vi "InVivoComputationalCannulaMicroscopeVi_v3.vi"() -> ()   [LabVIEW 2016]
doc: "The Grab and Attributes Setup example VI allows the user to view the current attributes and settings, update attribute settings, acquire images continuously, and display the images in an image control."
uses:
  <vilib>/Utility/error.llb/DialogType.ctl
  IVCCM Software V2/LabView Library/APT/callback_Done.vi
  IVCCM Software V2/LabView Library/GlobalVariables.vi
  D:/amcamsdk.20210816/extras/labview/toupcam.dll
  <vilib>/vision/NI_Vision_Development_Module.lvlib
panel:
  out "imgPro":u8[][](graph)
  in  "Imaging status":u16
  out "Error Out Surf Prep 2":errorcluster
  out "Error Surf 2":errorcluster
  in  "Full Toup Resolution":bool
  out "Image 2":u8[][](graph) caption="Image"
  out "Image":u16[][](graph)
  in  "Camera Idx":i32
  in  "Color Plane":i32(ring)=1 items=["Red", "Green", "Blue", "Hue", "Saturation", "Luminance", "Value", "Intensity"]
  out "objRef":u8[][](graph)
  in  "HW Tab":T1(tab)
  in  "LightVoltage":dbl
  in  "LightValue (v)":bool
  in  "MG17MotorZ":refnum<k7>(container)
  in  "MG17MotorY":refnum<k7>(container)
  in  "MG17MotorX":refnum<k7>(container)
  in  "Light Off (0v)":bool
  in  "Light On (5v)":bool
  in  "Grab":bool
  in  "ExpoGain":u16(slide) scale=100.0..5000.0
  in  "Expotime (ms)":dbl(slide)=300.0 scale=0.1..3600000.0
  in  "Saturation":i32(slide) scale=0.0..255.0
  in  "Hue":i32(slide) scale=-180.0..180.0
  in  "Gamma":i32(slide) scale=20.0..180.0
  in  "Contrast":i32(slide) scale=-100.0..100.0
  in  "Brightness":i32(slide) scale=-64.0..64.0
  in  "Error":errorcluster
  in  "Expotime_Min":u32
  in  "Expotime_Max":u32
  in  "ExpoGain_Min":u16
  in  "ExpoGain_Max":u16
  in  "ExpoGain_def":u16
  in  "Expotime_def":u32
  in  "LED Power":dbl=0.5
  in  "Orca Crop 2048x2048":T2={"Horizontal Offset"=1100, "Vertical Offset"=900, "Horizontal Width"=700, "Vertical Width"=700}
  in  "Toup Crop 5440x3648":T2={"Horizontal Offset"=3300, "Vertical Offset"=1200, "Horizontal Width"=1200, "Vertical Width"=1200}
  out "Timestamp":dbl
  out "Frames Per Second":dbl
  out "Library Version":string
  out "DCAM Version":string
  out "Error Cal":errorcluster
  in  "Z Index":i32=1
  out "Error Out Wait":errorcluster
  out "Error Surf":errorcluster
  out "Error Out Surf Prep":errorcluster
  out "Moving...":bool
  out "Saving...":bool
  in  "Pause":bool
  in  "Play":bool
  in  "Single":bool caption="Blank Button"
  in  "Load Cal":bool
  in  "Save Data":bool
  in  "Tab Control":T3(tab)
  in  "Stop Realtime\npix2pix":bool
  in  "Start Realtime\npix2pix":bool
  in  "Orca Exposure":dbl=3.0
  in  "Masking":bool
  in  "Threshold":dbl(slide) min=0.0 max=1.0 step=0.05 scale=0.0..1.0
  in  "Brigtness":dbl(slide) min=0.0 max=1.0 step=0.05 scale=0.0..1.0
  in  "Ctrl Factor":dbl(slide)=0.1 caption="Vertical Pointer Slide" min=0.0 max=100.0 step=0.01 scale=0.01..100.0
  in  "Shift input X":dbl step=1.0 format="%#.6g"
  in  "Shift Y":dbl step=1.0
  in  "Gain":dbl(slide)=1.0 min=1.0 step=0.05 scale=1.0..5.0
  in  "Convolution":bool
  in  "Frame Ave Count":dbl=1.0 min=0.0 max=1.0
  in  "Method":enum16{"Tikhonov", "DBS", "TSVD"}(ring)
  in  "Workspace":path=path "C:/Hun/Data/Calibration"
  in  "Kinetic Series":bool
  in  "Mask size (%)":i32=100 min=10 max=100 step=1
  in  "Mask Shift X":i32
  in  "Mask Shift Y":i32
  in  "Save image for pix2pix":bool
  in  "Z Retreat Pos":dbl
  in  "Z Retreat":bool
  in  "CalWait (ms)":dbl=60000.0
  in  "CalRepeat":dbl=1.0
  out "Cal Count":dbl
  in  "Wait (ms)":dbl
  in  "Z count":i32=1
  out "X Pos (mm)":sgl
  in  "X init":dbl=13.0
  in  "X size":dbl=0.02
  in  "Y count":i32=64
  in  "X count":i32=64
  in  "Start Cal":bool
  in  "Abort":bool
  out "Calibrating...":bool=TRUE
  in  "Calibration Folder":path=path "C:/Cannula Microscope/test"
  out "Y Pos (mm)":sgl
  out "Z Pos (mm)":sgl
  in  "Z size":dbl
  in  "Y size":dbl=0.02
  in  "Y init":dbl=13.0
  in  "Z init":dbl=4.68
  out "CalculatedRate":dbl
  in  "Calculate Shrink":bool
  out "Start Time":timestamp
  in  "Binning":dbl=1.0
  in  "StartShrinking":bool
  in  "FrameAve":dbl=1.0
  in  "Shrink":dbl
  out "lenSurface":dbl
  out "Count":dbl
  in  "Generate Surface & Go":bool
  in  "Clear Support":bool
  in  "Update Support Graph":bool
  in  "Save Support":bool
  out "XY Graph":cluster{"Y":dbl[], "Y":dbl[]}[](graph)
  out "zPos 2":sgl
  out "xPos 2":sgl
  out "yPos 2":sgl
  out "PointNumber":dbl
  out "Calibrating... 2":bool=TRUE
  out "Moving... 2":bool
  out "Saving... 2":bool
  in  "Abort 2":bool
  in  "Wait (ms) 2":dbl
  out "X Pos (mm) 2":sgl
  out "Y Pos (mm) 2":sgl
  out "Z Pos (mm) 2":sgl
  in  "ShrinkRate(mm/day)":dbl
  in  "Z Interval (mm)":dbl=0.005
  in  "Z depth (int)":dbl=19.0
  in  "FrameAve2":dbl=8.0
  in  "TimeZ":dbl
  in  "TimeY":dbl
  in  "TimeX":dbl
  in  "TimeFrames":dbl=10000.0
  out "Moving... 3":bool
  out "Capturing":bool
  out "X Pos (mm) 3":sgl
  out "Y Pos (mm) 3":sgl
  out "Count 2":dbl
  out "Z Pos (mm) 3":sgl
  in  "Abort 3":bool
  in  "Start Timelapse":bool
  in  "Time Interval":dbl=10000.0
  in  "FocusUp":bool
  in  "FocusDown":bool
  out "yPos":sgl
  out "xPos":sgl
  out "zPos":sgl
  in  "Down":bool
  in  "Up":bool
  in  "Right":bool
  in  "Left":bool
  in  "Stop":bool
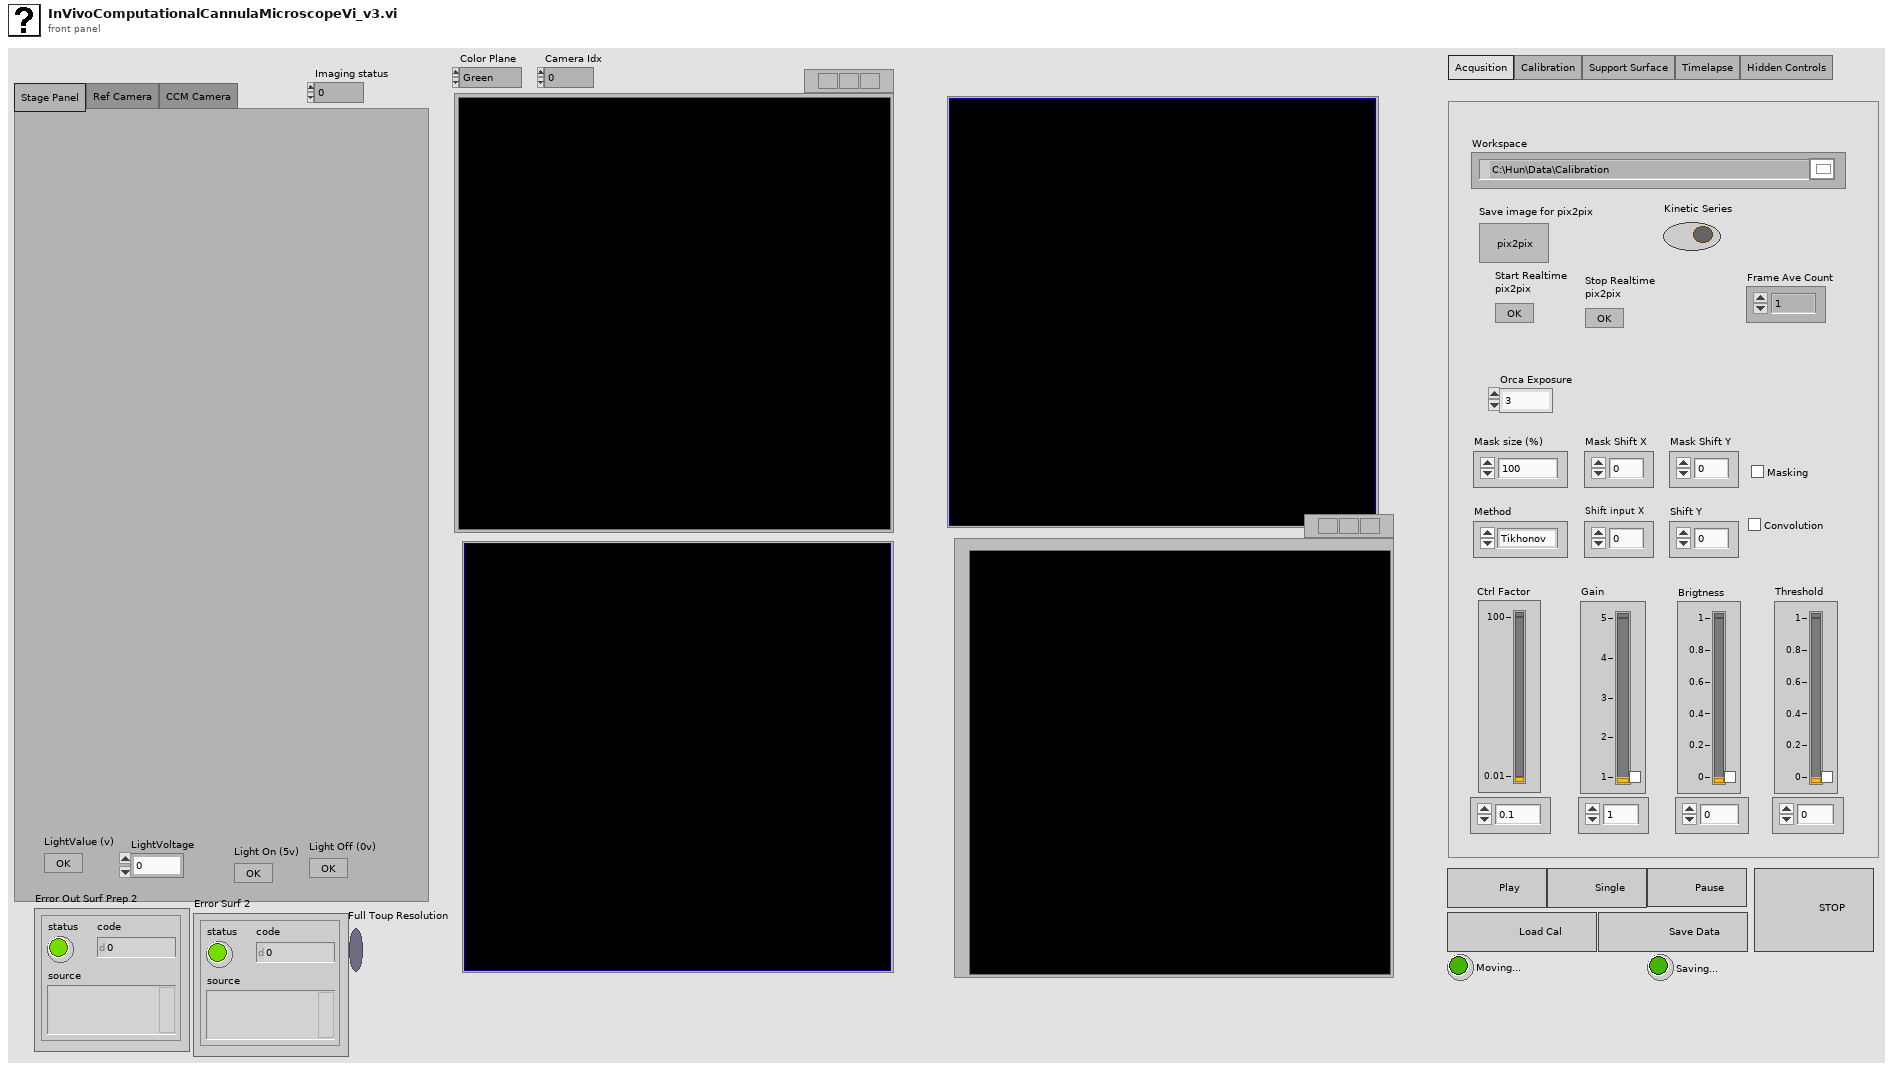
[diagram p1: front panel]
types:
  T1 = enum32{"Stage Panel", "Ref Camera", "CCM Camera"}
  T2 = cluster{"Horizontal Offset":i32, "Vertical Offset":i32, "Horizontal Width":i32, "Vertical Width":i32}
  T3 = enum32{"Acqusition", "Calibration", "Support Surface", "Timelapse", "Hidden Controls"}
  T4 = typedef "Image Type" = u32
  T5 = typedef "IMAQ Image.ctl" = refnum<image>
  T6 = typedef "DialogType.ctl" = u16
  T7 = cluster{"Capture Library":string, "DCAM-API":string}
  T8 = cluster{"height":u32, "width":u32, "datatype":u32}
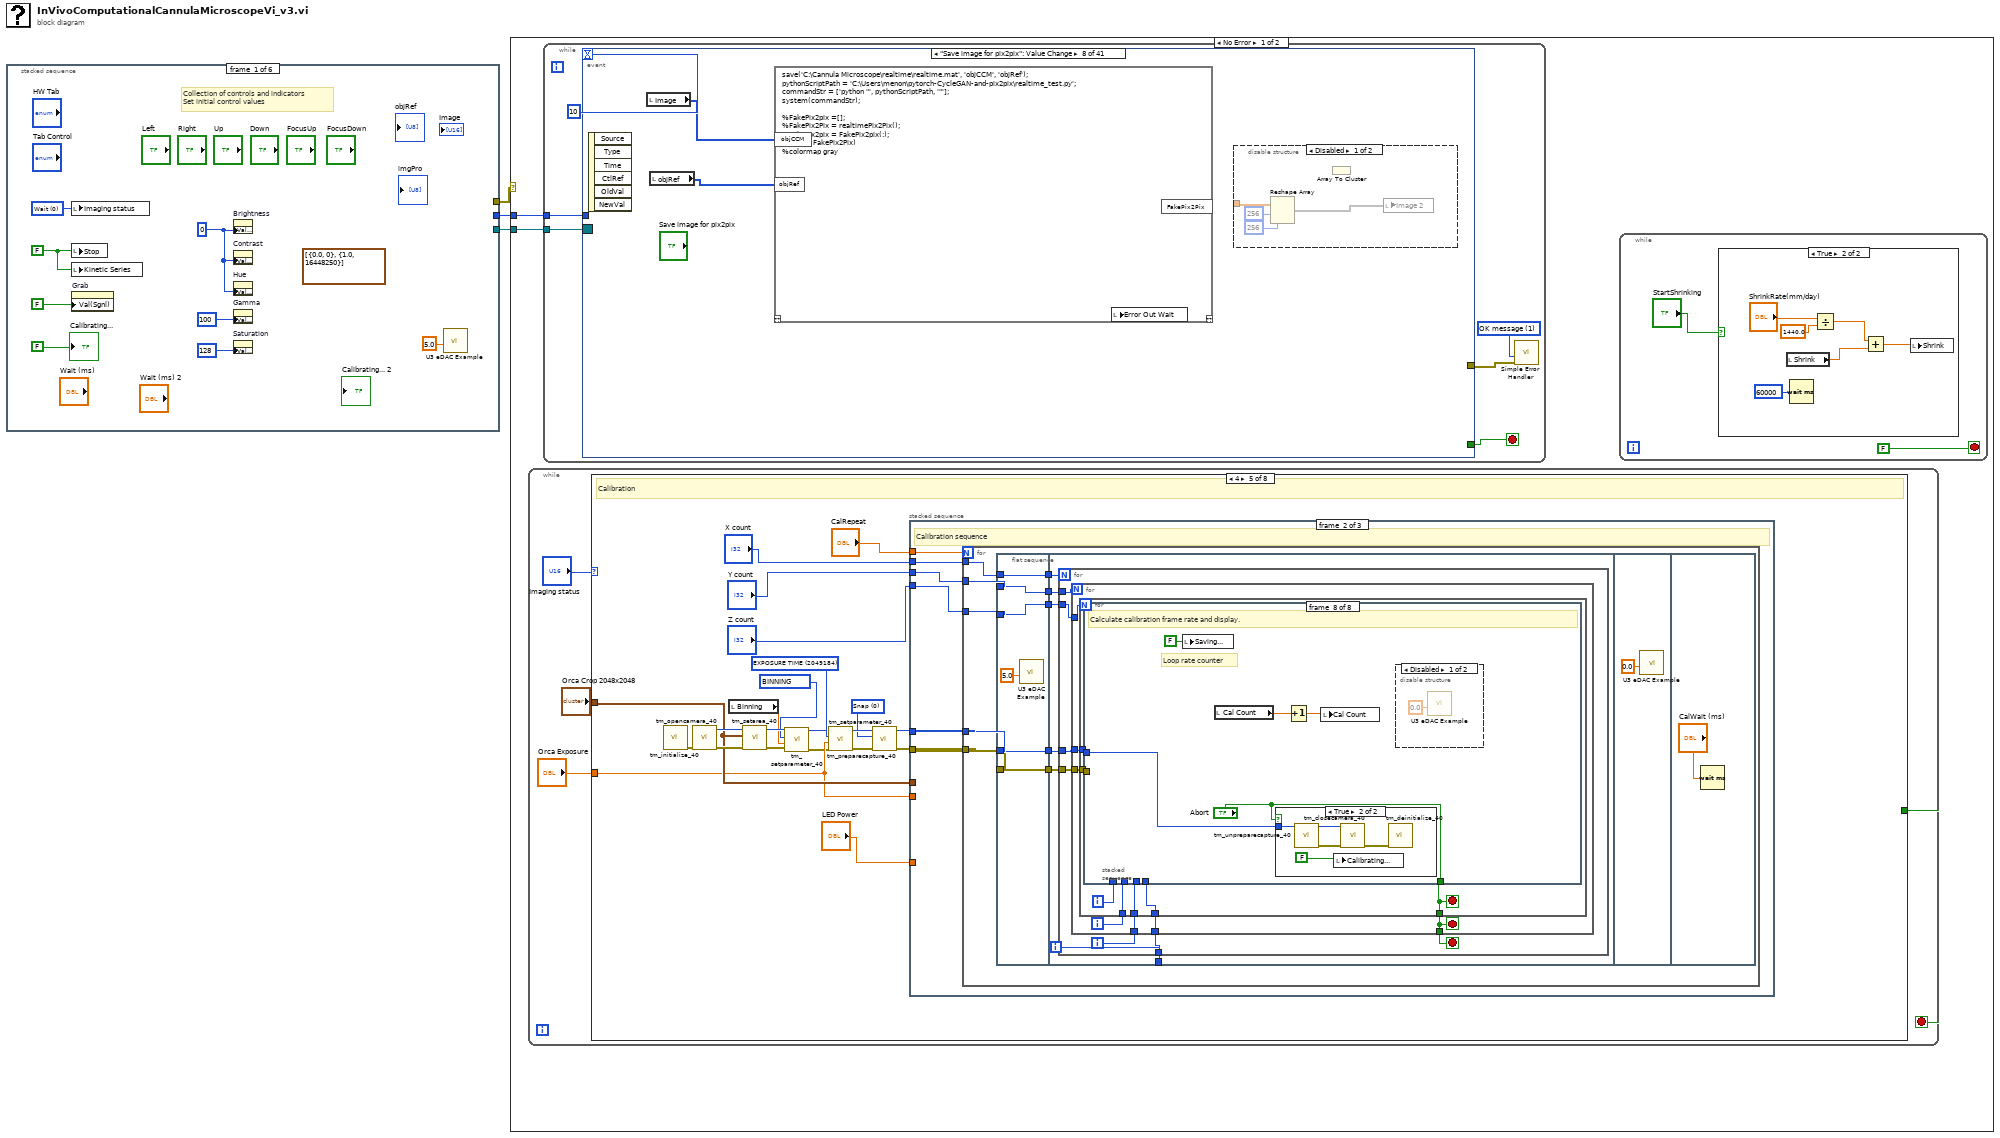
[diagram p0: block diagram]
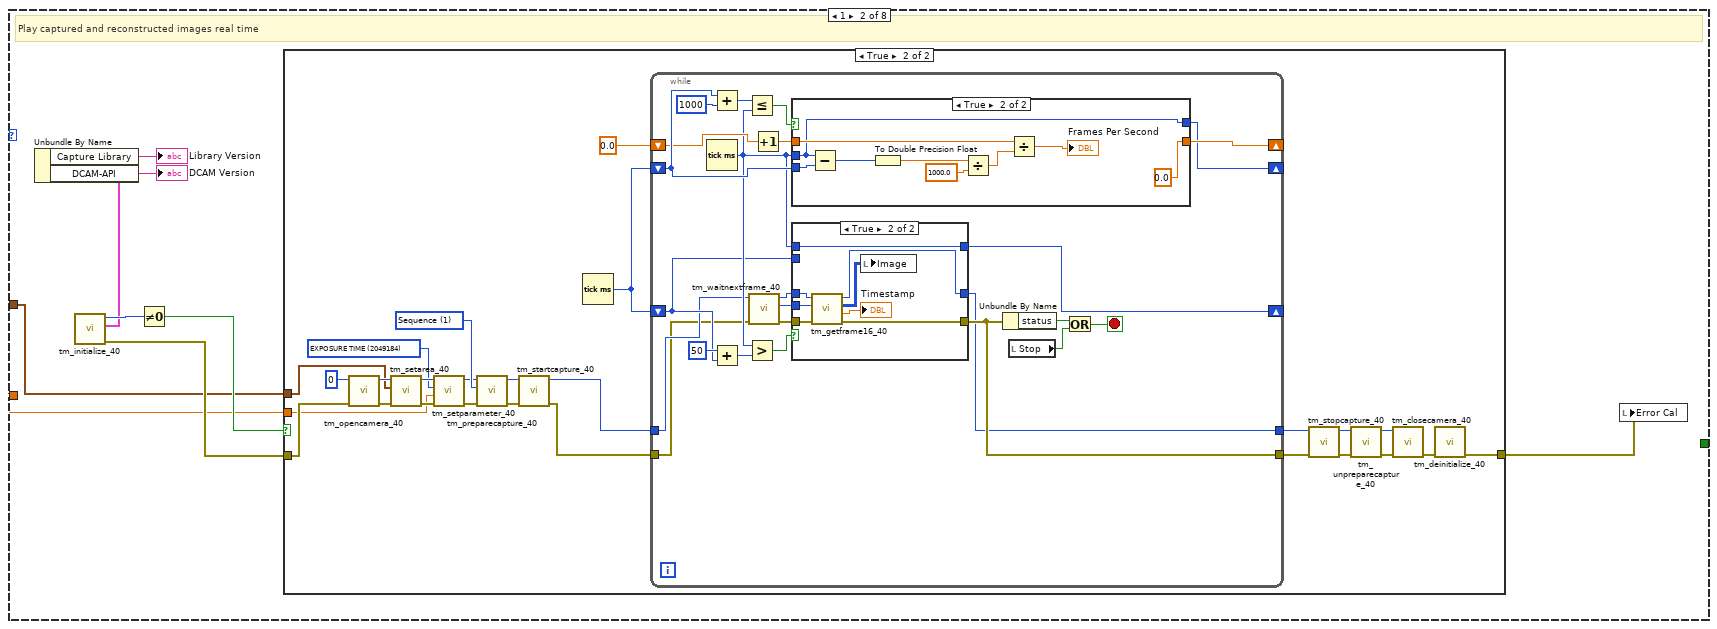
[diagram p4: hidden frame]
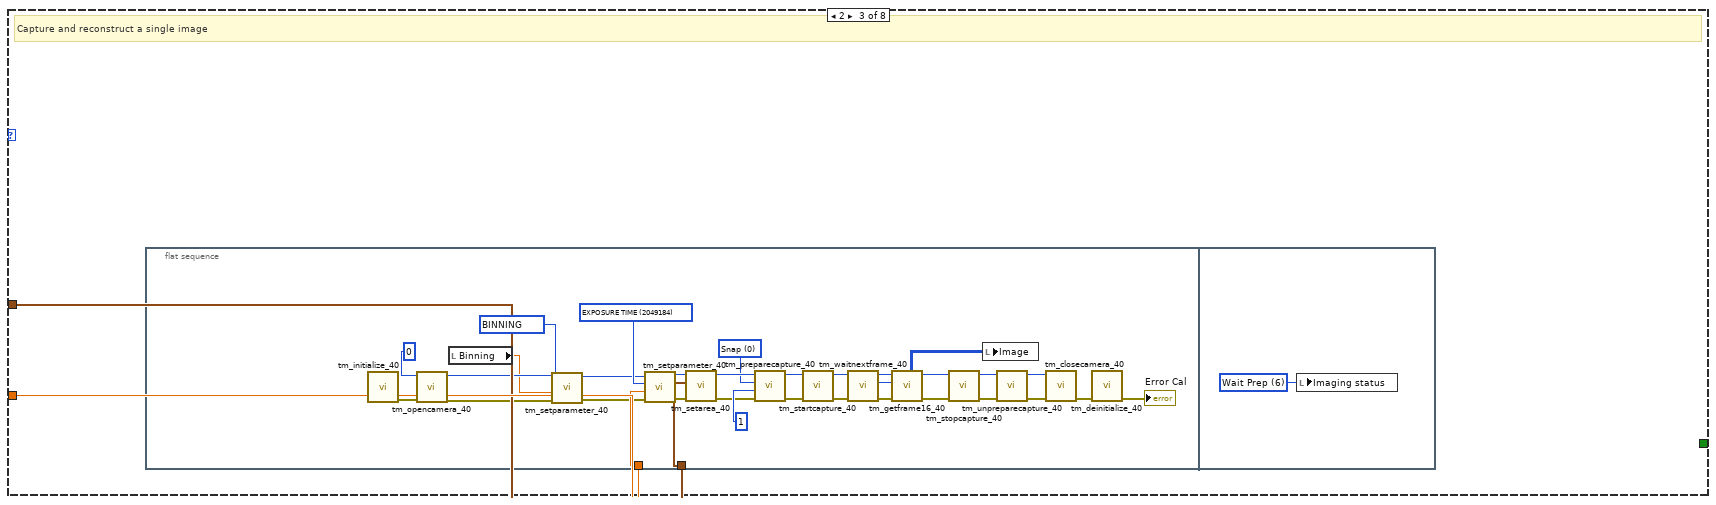
[diagram p8: hidden frame]
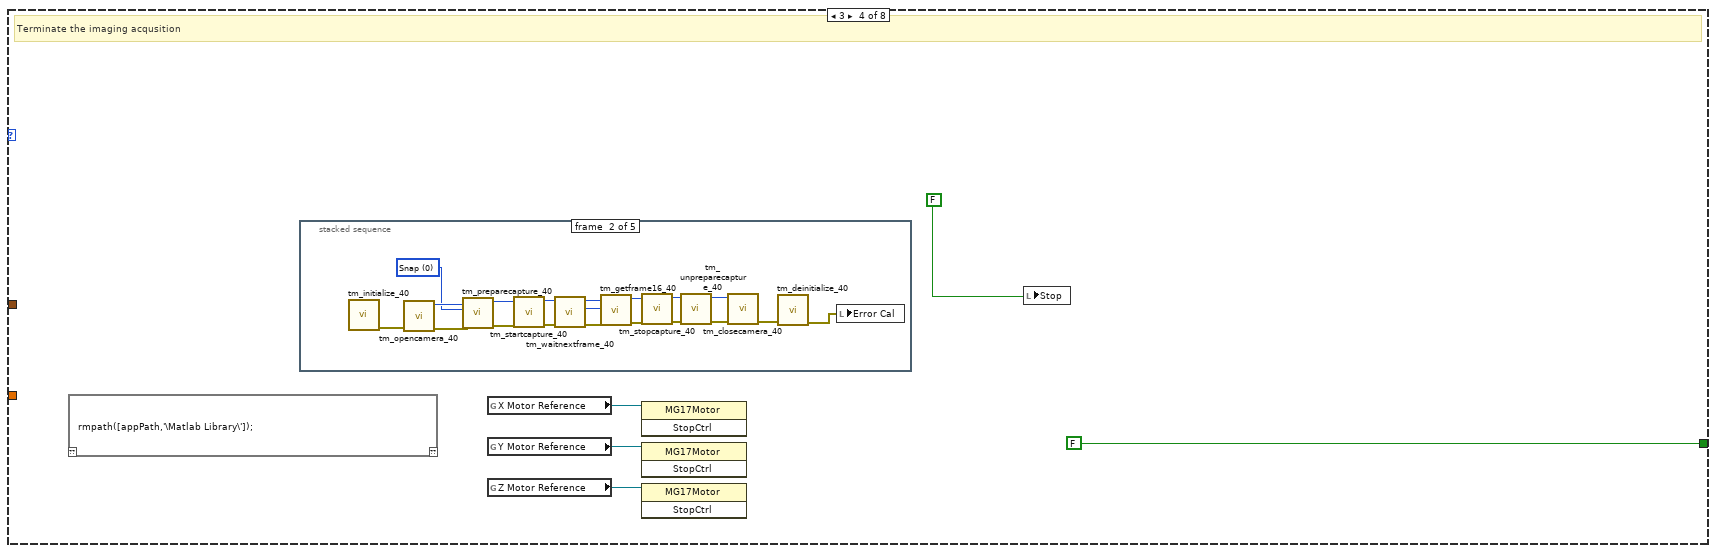
[diagram p9: hidden frame]
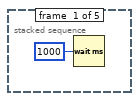
[diagram p10: hidden frame]
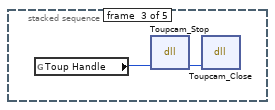
[diagram p11: hidden frame]
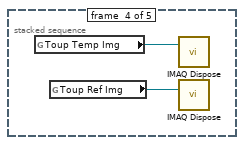
[diagram p12: hidden frame]
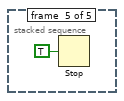
[diagram p13: hidden frame]
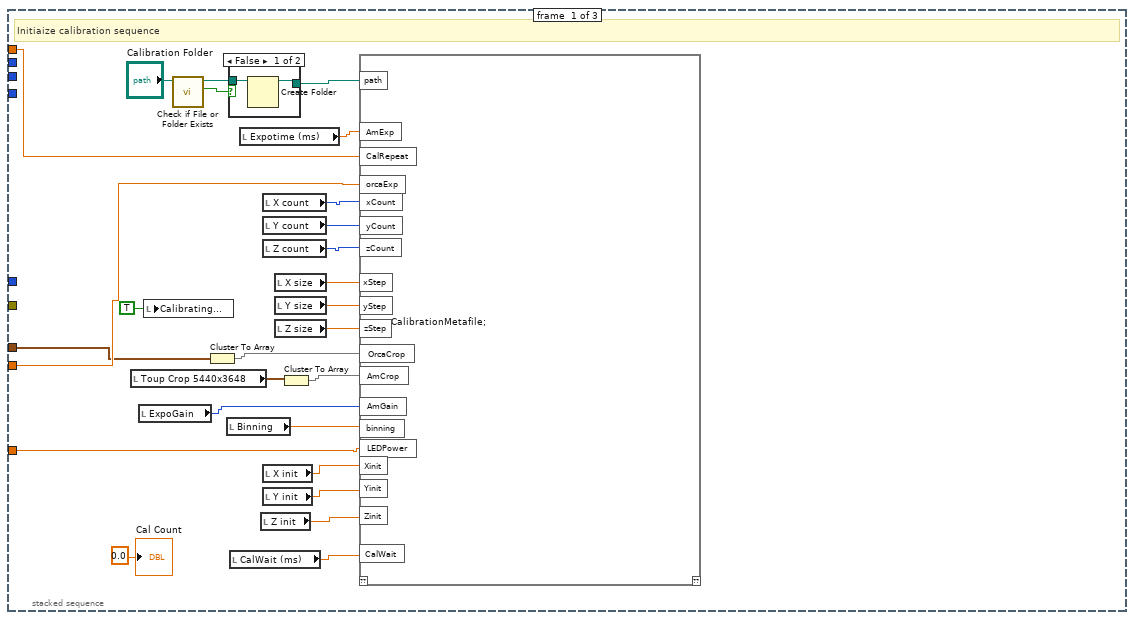
[diagram p14: hidden frame]
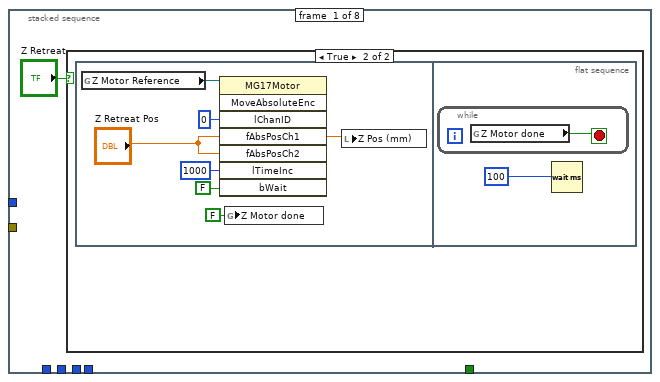
[diagram p16: hidden frame]
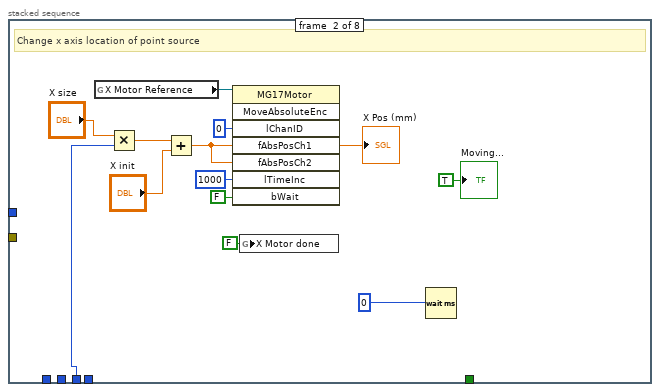
[diagram p18: hidden frame]
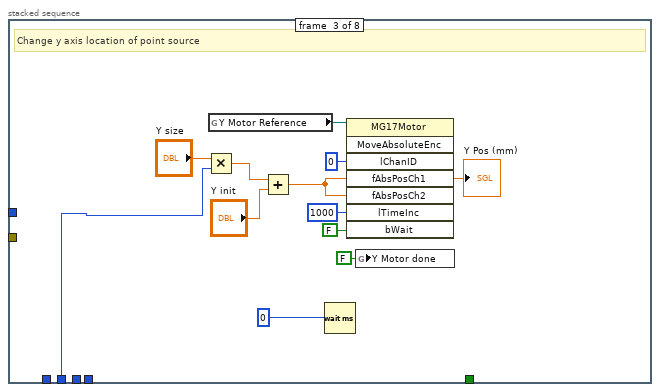
[diagram p19: hidden frame]
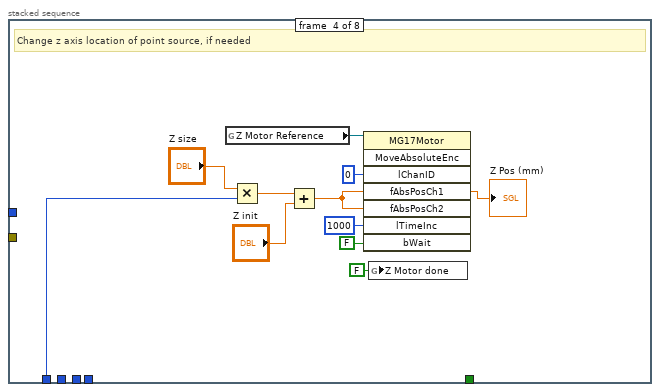
[diagram p20: hidden frame]
diagram:
  n1 = stacked-sequence {
    tunnel: [_ _ _ _ _ "Error"] -> w3
    tunnel: [_ _ w33 _ _ _] -> w2
    tunnel: [_ _ w32 _ _ _] -> w1
    frame #0 {
      w7 = 0
      (unwired) cluster{dbl, u32}[] [{0.0, 0}, {1.0, 16448250}] ("Z Scale.Marker Values[]")
      w9 = FALSE ("Stop")
      w10 = u16 0 items=["Wait", "Acquire Live", "Acquire Single", "Terminate"] ("Imaging status")
      # "Collection of controls and indicators\nSet initial control values"
      n2 = local write "Imaging status"(w10) -> ()
      n3 = local write "Stop"(w9) -> ()
      n4 = local write "Kinetic Series"(w9) -> ()
      n5 = property on="Grab" class="Bool (strict)"("Val(Sgnl)"=FALSE ("Value (Signaling)")) -> ()  [unwired: 2 in, 2 out]
      n6 = property on="Brightness" class="Slide (严格)"("Value"=w7) -> ()  [unwired: 2 in, 2 out]
      n7 = property on="Contrast" class="Slide (严格)"("Value"=w7) -> ()  [unwired: 2 in, 2 out]
      n8 = property on="Hue" class="Slide (严格)"("Value"=w7) -> ()  [unwired: 2 in, 2 out]
      n9 = property on="Gamma" class="Slide (严格)"("Value"=100) -> ()  [unwired: 2 in, 2 out]
      n10 = property on="Saturation" class="Slide (严格)"("Value"=128) -> ()  [unwired: 2 in, 2 out]
      n11 = call <userlib>:"U3 eDAC Example.vi"("Voltage"=5.0) -> ()  [unwired: 10 in, 1 out]
      "Calibrating..." <- FALSE
    }
    frame #1 {
      # "Initialize and configure motion control device, if any"
      n12 = vi-ref "callback_X.vi"() -> ("vi reference"=w17:refnum<vi>)
      n13 = vi-ref "callback_Y.vi"() -> ("vi reference"=w20:refnum<vi>)
      n14 = vi-ref "callback_Z.vi"() -> ("vi reference"=w21:refnum<vi>)
      n15 = call "initializeStage.vi"("VI Ref"=w17, "HWSerialNum"=83845474, "reference"="MG17MotorX") -> ("reference out"=w14:refnum<k7>)  [unwired: 8 in]
      n16 = call "initializeStage.vi"("VI Ref"=w20, "HWSerialNum"=83841126, "reference"="MG17MotorY") -> ("reference out"=w13:refnum<k7>)  [unwired: 8 in]
      n17 = call "initializeStage.vi"("VI Ref"=w21, "HWSerialNum"=49864805, "reference"="MG17MotorZ") -> ("reference out"=w12:refnum<k7>)  [unwired: 8 in]
      n18 = global write "callback_Done.vi" "X Motor Reference"(w14) -> ()
      n19 = global write "callback_Done.vi" "Y Motor Reference"(w13) -> ()
      n20 = global write "callback_Done.vi" "Z Motor Reference"(w12) -> ()
    }
    frame #2 {
      w25 = u32 1000 ("y")
      w38 = T4 4 items=["Grayscale (U8)", "Grayscale (I16)", "Grayscale (SGL)", "Complex (CSG)", "RGB (U32)", "HSL (U32)", "RGB (U64)", "Grayscale (U16)"] ("Image Type")
      # "SetSliderRange"
      n21 = call "init.vi"("Camera Idx"="Camera Idx") -> ("Event Registration Refnum"=w33:refnum<event-registration>, "htoupcam"=w32:i32, "Cluster"=w37:cluster{"pWidth":i32, "pHeight":i32})  [unwired: 8 in]
      n22 = global write "GlobalVariables.vi" "Toup Event"(w33) -> ()
      n23 = global write "GlobalVariables.vi" "Toup Resolution"(w37) -> ()
      n24 = global write "GlobalVariables.vi" "Toup Handle"(w32) -> ()
      n25 = dll-call lib="D:/amcamsdk.20210816/extras/labview/toupcam.dll" fn="Toupcam_get_ExpTimeRange"("htoupcam"=w32, "nMin"="Expotime_Min", "nMax"="Expotime_Max", "ndef"="Expotime_def") -> ("nMin"=w31:u32, "nMax"=w29:u32, "ndef"=w27:u32)  [unwired: 5 in, 2 out]
      n26 = dll-call lib="D:/amcamsdk.20210816/extras/labview/toupcam.dll" fn="Toupcam_get_ExpoAGainRange"("htoupcam"=w32, "nmin"="ExpoGain_Min", "nmax"="ExpoGain_Max", "ndef"="ExpoGain_def") -> ("nmin"=w46:u16, "nmax"=w45:u16, "ndef"=w44:u16)  [unwired: 5 in, 2 out]
      n27 = property on="ExpoGain" class="Slide (严格)"("Scale.Minimum"=w46, "Scale.Maximum"=w45, "Value"=w44) -> ()  [unwired: 2 in, 2 out]
      n28 = Divide(x=w31, y=w25) -> (x/y=w30:dbl)
      n29 = Divide(x=w29, y=w25) -> (x/y=w28:dbl)
      n30 = Divide(x=w27, y=w25) -> (x/y=w26:dbl)
      n31 = property on="Expotime (ms)" class="Slide (strict)"("Scale.Minimum"=w30, "Scale.Maximum"=w28, "Value"=w26) -> ()  [unwired: 2 in, 2 out]
      n32 = call "IMAQ Create"("Image Name"="refImg") -> ("New Image"=w34:T5)  [unwired: 4 in, 1 out]
      n33 = call "IMAQ Create"("Image Name"="tempImg", "Image Type"=w38) -> ("New Image"=w35:T5)  [unwired: 3 in, 1 out]
      n34 = global write "GlobalVariables.vi" "Toup Ref Img"(w34) -> ()
      n35 = global write "GlobalVariables.vi" "Toup Temp Img"(w35) -> ()
    }
    frame #3 {
      w56 = T6 1 items=["no dialog", "OK message", "continue or stop message", "OK message + warnings", "continue/stop + warnings"] ("type of dialog (OK msg:1)")
      # "Initialize Matlab variables with initial control values"
      n36 = local read "Orca Exposure"() -> (w49:dbl)
      n37 = local read "Mask size (%)"() -> (w53:i32)
      n38 = local read "Convolution"() -> (w60:bool)
      n39 = local read "Mask Shift X"() -> (w52:i32)
      n40 = local read "Mask Shift Y"() -> (w51:i32)
      n41 = local read "Ctrl Factor"() -> (w67:dbl)
      n42 = local read "Threshold"() -> (w62:dbl)
      n43 = local read "Shift input X"() -> (w65:dbl)
      n44 = local read "Brigtness"() -> (w63:dbl)
      n45 = local read "Masking"() -> (w54:bool)
      n46 = local read "Method"() -> (w59:enum16{"Tikhonov", "DBS", "TSVD"})
      n47 = local read "Z Index"() -> (w50:i32)
      n48 = local read "Shift Y"() -> (w66:dbl)
      n49 = local read "Gain"() -> (w64:dbl)
      n50 = call <vilib>:"Application Directory.vi"() -> ("Application Directory"=w58:path)
      n51 = Boolean To (0,1)(Boolean=w54) -> (0, 1=w55:i16)
      n52 = Boolean To (0,1)(Boolean=w60) -> (0, 1=w61:i16)
      n53 = script code="addpath([appPath,'\\Matlab Library\\']);\n\nzSize = 1;\nDC = 0;\npsfSize = 111;\nnormArray = ones(psfSize,psfSize);\n\nxPos = 0;\nyPos = 0;\nzPos = 0;\nimgRaw = 0;\nobjRef = 0;\n\nzInd = 1;\nf = 1;\nsaveMode = 'single';\nsaveObjPro = false;\nsaveImgPro = false;\ninitFrame;"("sfX"=w65, "sfY"=w66, "ctrlFactor"=w67, "method"=w59, "threshold"=w62, "brightness"=w63, "gain"=w64, "convOpt"=w61, "appPath"=w58, "maskOpt"=w55, "maskSize"=w53, "maskShiftX"=w52, "maskShiftY"=w51, "zInd"=w50, "Exp"=w49) -> ("??"=w57:errorcluster)  [unwired: 1 in]
      n54 = call <vilib>:"Simple Error Handler.vi"("type of dialog (OK msg:1)"=w56, "error in (no error)"=w57) -> ()  [unwired: 3 in, 5 out]
    }
    frame #4 {
      n55 = disable-structure shown="Enabled" {
        frame Disabled {
          w70 = T6 1 items=["no dialog", "OK message", "continue or stop message", "OK message + warnings", "continue/stop + warnings"] ("type of dialog (OK msg:1)")
          n56 = local read "Mask Shift Y"() -> (w68:i32)
          n57 = script code="test=999;"("maskShiftY"=w68) -> ("??"=w69:errorcluster)  [unwired: 1 in]
          n58 = call <vilib>:"Simple Error Handler.vi"("type of dialog (OK msg:1)"=w70, "error in (no error)"=w69) -> ()  [unwired: 3 in, 5 out]
        }
        frame Enabled {
        }
      }
    }
    frame #5 {
    }
  }
  n59 = case shown="No Error" w3 {
    selector: w3 -> [_ w993]
    tunnel: w2 -> [w73 _]
    tunnel: w1 -> [w72 _]
    frame No Error {
      n60 = while {
        stop <- w85 stop-if-true
        n61 = case shown="4" "Imaging status" {
          tunnel: [_ _ _ FALSE _ _ _ _] -> w85
          tunnel: "Orca Crop 2048x2048" -> [_ w88 w168 _ w251 w448 w588 _]
          tunnel: "Orca Exposure" -> [_ w87 w169 _ w249 w447 w587 _]
          frame 0, Default {
            # "Wait"
          }
          frame 1 {
            # "Play captured and reconstructed images real time"
            n62 = call <userlib>:"tm_initialize_40.vi"() -> ("error out"=w92:errorcluster, "Version Info"=w91:T7, "Number Of Cameras"=w93:u32)  [unwired: 8 in, 1 out]
            n63 = Unbundle By Name(w91) -> ("Capture Library"=→"Library Version":string, "DCAM-API"=→"DCAM Version":string)
            n64 = Not Equal To 0?(x=w93) -> (x != 0?=w94:bool)
            n65 = case shown="True" w94 {
              tunnel: w92 -> [w95 w121]
              tunnel: [w95 w105] -> w86
              tunnel: w88 -> [_ w97]
              tunnel: w87 -> [_ w96]
              frame False {
              }
              frame True {
                w102 = u32 2049184 items=["SENSOR MODE"=4212128, "READOUT SPEED"=4211872, "READOUT DIRECTION"=4211904, "TRIGGER GLOBAL EXPOSURE"=2049680, "TRIGGER DELAY"=1066480, "INTERNAL TRIGGER HANDLING"=1066496, "SYNC READOUT SYSTEM BLANK"=1066528, "SENSOR TEMPERATURE"=2115232, "SENSOR COOLER STATUS"=2115280, "EXPOSURE TIME"=2049184, "DEFECT CORRECT MODE"=4670368, "BINNING"=4215968, "INTERNAL LINE SPEED"=4226000, "INTERNAL LINE INTERVAL"=4226016, "NUMBER OF OUTPUT TRIGGER CONNECTOR"=1852320, "OUTPUT TRIGGER SOURCE[0]"=1852576, "OUTPUT TRIGGER SOURCE[1]"=1852832, "OUTPUT TRIGGER SOURCE[2]"=1853088, "OUTPUT TRIGGER POLARITY[0]"=1852592, "OUTPUT TRIGGER POLARITY[1]"=1852848, "OUTPUT TRIGGER POLARITY[2]"=1853104, "OUTPUT TRIGGER ACTIVE[0]"=1852608, "OUTPUT TRIGGER ACTIVE[1]"=1852864, "OUTPUT TRIGGER ACTIVE[2]"=1853120, "OUTPUT TRIGGER DELAY[0]"=1852624, "OUTPUT TRIGGER DELAY[1]"=1852880, "OUTPUT TRIGGER DELAY[2]"=1853136, "OUTPUT TRIGGER PERIOD[0]"=1852640, "OUTPUT TRIGGER PERIOD[1]"=1852896, "OUTPUT TRIGGER PERIOD[2]"=1853152, "OUTPUT TRIGGER KIND[0]"=1852656, "OUTPUT TRIGGER KIND[1]"=1852912, "OUTPUT TRIGGER KIND[2]"=1853168, "OUTPUT TRIGGER BASE SENSOR[0]"=1852672, "OUTPUT TRIGGER BASE SENSOR[1]"=1852928, "OUTPUT TRIGGER BASE SENSOR[2]"=1853184, "OUTPUT TRIGGER PRE HSYNC COUNT"=1852704] ("Parameter")
                w111 = 1 items=["Snap", "Sequence"] ("Capture mode")
                n66 = call <userlib>:"tm_opencamera_40.vi"("error in (no error)"=w121, "Camera Index"=u32 0) -> ("error out"=w100:errorcluster, "Handle out"=w101:u32)  [unwired: 7 in, 1 out]
                n67 = call <userlib>:"tm_setarea_40.vi"("error in (no error)"=w100, "Sub Region"=w97, "Handle in"=w101) -> ("error out"=w103:errorcluster, "Handle out"=w104:u32)  [unwired: 7 in]
                n68 = call <userlib>:"tm_setparameter_40.vi"("error in (no error)"=w103, "Value in"=w96, "Parameter"=w102, "Handle in"=w104) -> ("error out"=w98:errorcluster, "Handle out"=w99:u32)  [unwired: 6 in]
                n69 = call <userlib>:"tm_preparecapture_40.vi"("error in (no error)"=w98, "Capture mode"=w111, "Handle in"=w99) -> ("error out"=w109:errorcluster, "Handle out"=w110:u32)  [unwired: 5 in, 2 out]
                n70 = call <userlib>:"tm_startcapture_40.vi"("error in (no error)"=w109, "Handle in"=w110) -> ("error out"=w112:errorcluster, "Handle out"=w113:u32)  [unwired: 8 in]
                n71 = Tick Count (ms)() -> (millisecond timer value=w107:u32)
                n72 = while {
                  tunnel: [w127] -> w116
                  tunnel: [w128] -> w117
                  tunnel: w113 -> [w124]
                  tunnel: w112 -> [w123]
                  shift-right: [w143] -> _
                  shift-left: w107 -> [w140]
                  shift-right: [w144] -> _
                  shift-left: 0.0 -> [w137]
                  shift-right: [w126] -> _
                  shift-left: w107 -> [w129]
                  stop <- w125 stop-if-true
                  n73 = Tick Count (ms)() -> (millisecond timer value=w130:u32)
                  n74 = Add(x=w140, y=u32 1000) -> (x+y=w142:u32)
                  n75 = Add(x=u32 50, y=w129) -> (x+y=w132:u32)
                  n76 = Less Or Equal?(x=w142, y=w130) -> (x <= y?=w139:bool)
                  n77 = Greater?(x=w130, y=w132) -> (0:w131:bool)
                  n78 = call <userlib>:"tm_waitnextframe_40.vi"("error in (no error)"=w123, "Handle in"=w124) -> ("error out"=w135:errorcluster, "Frame Index"=w134:i32, "Handle out"=w136:u32)  [unwired: 6 in, 1 out]
                  n79 = Increment(x=w137) -> (x+1=w138:dbl)
                  n80 = case shown="True" w139 {
                    tunnel: w140 -> [w158 w161]
                    tunnel: [w158 w159] -> w143
                    tunnel: w138 -> [w157 w165]
                    tunnel: w130 -> [_ w159]
                    tunnel: [w157 0.0] -> w144
                    frame False {
                    }
                    frame True {
                      n81 = Subtract(x=w159, y=w161) -> (x-y=w160:u32)
                      n82 = To Double Precision Float(number=w160) -> (double precision float=w167:dbl)
                      n83 = Divide(x=w167, y=1000.0) -> (x/y=w164:dbl)
                      n84 = Divide(x=w165, y=w164) -> (x/y=→"Frames Per Second":dbl)
                    }
                  }
                  n85 = case shown="True" w131 {
                    tunnel: w136 -> [w148 w156]
                    tunnel: w135 -> [w147 w155]
                    tunnel: w134 -> [_ w150]
                    tunnel: w129 -> [w146 _]
                    tunnel: w130 -> [_ w154]
                    tunnel: [w148 w152] -> w127
                    tunnel: [w147 w153] -> w128
                    tunnel: [w146 w154] -> w126
                    frame False {
                    }
                    frame True {
                      n86 = call <userlib>:"tm_getframe16_40.vi"("error in (no error)"=w155, "Frame Index"=w150, "Handle in"=w156) -> ("error out"=w153:errorcluster, "Timestamp"=→"Timestamp":dbl, "Data"=w149:u16[][], "Handle out"=w152:u32)  [unwired: 5 in]
                      n87 = local write "Image"(w149) -> ()
                    }
                  }
                  n88 = Unbundle By Name(w128) -> ("status"=w145:bool)
                  n89 = local read "Stop"() -> (w122:bool)
                  n90 = Or(x=w145, y=w122) -> (x .or. y?=w125:bool)
                }
                n91 = call <userlib>:"tm_stopcapture_40.vi"("error in (no error)"=w117, "Handle in"=w116) -> ("error out"=w114:errorcluster, "Handle out"=w115:u32)  [unwired: 8 in]
                n92 = call <userlib>:"tm_unpreparecapture_40.vi"("error in (no error)"=w114, "Handle in"=w115) -> ("error out"=w119:errorcluster, "Handle out"=w118:u32)  [unwired: 8 in]
                n93 = call <userlib>:"tm_closecamera_40.vi"("error in (no error)"=w119, "Handle in"=w118) -> ("error out"=w106:errorcluster)  [unwired: 9 in]
                n94 = call <userlib>:"tm_deinitialize_40.vi"("error in (no error)"=w106) -> ("error out"=w105:errorcluster)  [unwired: 10 in]
              }
            }
            n95 = local write "Error Cal"(w86) -> ()
          }
          frame 2 {
            # "Capture and reconstruct a single image"
            n96 = flat-sequence {
              tunnel: w169 -> [w202]
              tunnel: w168 -> [w201]
              frame #0 {
                w171 = u32 4215968 items=["SENSOR MODE"=4212128, "READOUT SPEED"=4211872, "READOUT DIRECTION"=4211904, "TRIGGER GLOBAL EXPOSURE"=2049680, "TRIGGER DELAY"=1066480, "INTERNAL TRIGGER HANDLING"=1066496, "SYNC READOUT SYSTEM BLANK"=1066528, "SENSOR TEMPERATURE"=2115232, "SENSOR COOLER STATUS"=2115280, "EXPOSURE TIME"=2049184, "DEFECT CORRECT MODE"=4670368, "BINNING"=4215968, "INTERNAL LINE SPEED"=4226000, "INTERNAL LINE INTERVAL"=4226016, "NUMBER OF OUTPUT TRIGGER CONNECTOR"=1852320, "OUTPUT TRIGGER SOURCE[0]"=1852576, "OUTPUT TRIGGER SOURCE[1]"=1852832, "OUTPUT TRIGGER SOURCE[2]"=1853088, "OUTPUT TRIGGER POLARITY[0]"=1852592, "OUTPUT TRIGGER POLARITY[1]"=1852848, "OUTPUT TRIGGER POLARITY[2]"=1853104, "OUTPUT TRIGGER ACTIVE[0]"=1852608, "OUTPUT TRIGGER ACTIVE[1]"=1852864, "OUTPUT TRIGGER ACTIVE[2]"=1853120, "OUTPUT TRIGGER DELAY[0]"=1852624, "OUTPUT TRIGGER DELAY[1]"=1852880, "OUTPUT TRIGGER DELAY[2]"=1853136, "OUTPUT TRIGGER PERIOD[0]"=1852640, "OUTPUT TRIGGER PERIOD[1]"=1852896, "OUTPUT TRIGGER PERIOD[2]"=1853152, "OUTPUT TRIGGER KIND[0]"=1852656, "OUTPUT TRIGGER KIND[1]"=1852912, "OUTPUT TRIGGER KIND[2]"=1853168, "OUTPUT TRIGGER BASE SENSOR[0]"=1852672, "OUTPUT TRIGGER BASE SENSOR[1]"=1852928, "OUTPUT TRIGGER BASE SENSOR[2]"=1853184, "OUTPUT TRIGGER PRE HSYNC COUNT"=1852704] ("Parameter")
                w183 = u32 2049184 items=["SENSOR MODE"=4212128, "READOUT SPEED"=4211872, "READOUT DIRECTION"=4211904, "TRIGGER GLOBAL EXPOSURE"=2049680, "TRIGGER DELAY"=1066480, "INTERNAL TRIGGER HANDLING"=1066496, "SYNC READOUT SYSTEM BLANK"=1066528, "SENSOR TEMPERATURE"=2115232, "SENSOR COOLER STATUS"=2115280, "EXPOSURE TIME"=2049184, "DEFECT CORRECT MODE"=4670368, "BINNING"=4215968, "INTERNAL LINE SPEED"=4226000, "INTERNAL LINE INTERVAL"=4226016, "NUMBER OF OUTPUT TRIGGER CONNECTOR"=1852320, "OUTPUT TRIGGER SOURCE[0]"=1852576, "OUTPUT TRIGGER SOURCE[1]"=1852832, "OUTPUT TRIGGER SOURCE[2]"=1853088, "OUTPUT TRIGGER POLARITY[0]"=1852592, "OUTPUT TRIGGER POLARITY[1]"=1852848, "OUTPUT TRIGGER POLARITY[2]"=1853104, "OUTPUT TRIGGER ACTIVE[0]"=1852608, "OUTPUT TRIGGER ACTIVE[1]"=1852864, "OUTPUT TRIGGER ACTIVE[2]"=1853120, "OUTPUT TRIGGER DELAY[0]"=1852624, "OUTPUT TRIGGER DELAY[1]"=1852880, "OUTPUT TRIGGER DELAY[2]"=1853136, "OUTPUT TRIGGER PERIOD[0]"=1852640, "OUTPUT TRIGGER PERIOD[1]"=1852896, "OUTPUT TRIGGER PERIOD[2]"=1853152, "OUTPUT TRIGGER KIND[0]"=1852656, "OUTPUT TRIGGER KIND[1]"=1852912, "OUTPUT TRIGGER KIND[2]"=1853168, "OUTPUT TRIGGER BASE SENSOR[0]"=1852672, "OUTPUT TRIGGER BASE SENSOR[1]"=1852928, "OUTPUT TRIGGER BASE SENSOR[2]"=1853184, "OUTPUT TRIGGER PRE HSYNC COUNT"=1852704] ("Parameter")
                w176 = 0 items=["Snap", "Sequence"] ("Capture mode")
                n97 = call <userlib>:"tm_initialize_40.vi"() -> ("error out"=w200:errorcluster)  [unwired: 8 in, 3 out]
                n98 = call <userlib>:"tm_opencamera_40.vi"("error in (no error)"=w200, "Camera Index"=u32 0) -> ("error out"=w172:errorcluster, "Handle out"=w175:u32)  [unwired: 7 in, 1 out]
                n99 = local read "Binning"() -> (w170:dbl)
                n100 = call <userlib>:"tm_setparameter_40.vi"("error in (no error)"=w172, "Value in"=w170, "Parameter"=w171, "Handle in"=w175) -> ("error out"=w173:errorcluster, "Handle out"=w174:u32)  [unwired: 6 in]
                n101 = call <userlib>:"tm_setparameter_40.vi"("error in (no error)"=w173, "Value in"=w202, "Parameter"=w183, "Handle in"=w174) -> ("error out"=w179:errorcluster, "Handle out"=w182:u32)  [unwired: 6 in]
                n102 = call <userlib>:"tm_setarea_40.vi"("error in (no error)"=w179, "Sub Region"=w201, "Handle in"=w182) -> ("error out"=w180:errorcluster, "Handle out"=w181:u32)  [unwired: 7 in]
                n103 = call <userlib>:"tm_preparecapture_40.vi"("error in (no error)"=w180, "Frames"=1, "Capture mode"=w176, "Handle in"=w181) -> ("error out"=w192:errorcluster, "Handle out"=w193:u32)  [unwired: 4 in, 2 out]
                n104 = call <userlib>:"tm_startcapture_40.vi"("error in (no error)"=w192, "Handle in"=w193) -> ("error out"=w190:errorcluster, "Handle out"=w189:u32)  [unwired: 8 in]
                n105 = call <userlib>:"tm_waitnextframe_40.vi"("error in (no error)"=w190, "Handle in"=w189) -> ("error out"=w188:errorcluster, "Frame Index"=w184:i32, "Handle out"=w187:u32)  [unwired: 6 in, 1 out]
                n106 = call <userlib>:"tm_getframe16_40.vi"("error in (no error)"=w188, "Frame Index"=w184, "Handle in"=w187) -> ("error out"=w185:errorcluster, "Data"=w178:u16[][], "Handle out"=w186:u32)  [unwired: 5 in, 1 out]
                n107 = call <userlib>:"tm_stopcapture_40.vi"("error in (no error)"=w185, "Handle in"=w186) -> ("error out"=w194:errorcluster, "Handle out"=w195:u32)  [unwired: 8 in]
                n108 = local write "Image"(w178) -> ()
                n109 = call <userlib>:"tm_unpreparecapture_40.vi"("error in (no error)"=w194, "Handle in"=w195) -> ("error out"=w197:errorcluster, "Handle out"=w196:u32)  [unwired: 8 in]
                n110 = call <userlib>:"tm_closecamera_40.vi"("error in (no error)"=w197, "Handle in"=w196) -> ("error out"=w198:errorcluster)  [unwired: 9 in]
                n111 = call <userlib>:"tm_deinitialize_40.vi"("error in (no error)"=w198) -> ("error out"=→"Error Cal":errorcluster)  [unwired: 10 in]
              }
              frame #1 {
                w203 = u16 6 items=["Wait", "Acquire Live", "Acquire Single", "Terminate", "Calibration", "Macro", "Wait Prep"] ("Imaging status")
                n112 = local write "Imaging status"(w203) -> ()
              }
            }
          }
          frame 3 {
            # "Terminate the imaging acqusition"
            n113 = script code="rmpath([appPath,'\\Matlab Library\\']);"() -> ()  [unwired: 1 in, 1 out]
            n114 = stacked-sequence {
              frame #0 {
                n115 = Wait (ms)(milliseconds to wait=u32 1000) -> ()  [unwired: 1 out]
              }
              frame #1 {
                w215 = 0 items=["Snap", "Sequence"] ("Capture mode")
                n116 = call <userlib>:"tm_initialize_40.vi"() -> ("error out"=w227:errorcluster)  [unwired: 8 in, 3 out]
                n117 = call <userlib>:"tm_opencamera_40.vi"("error in (no error)"=w227) -> ("error out"=w226:errorcluster, "Handle out"=w220:u32)  [unwired: 8 in, 1 out]
                n118 = call <userlib>:"tm_preparecapture_40.vi"("error in (no error)"=w226, "Capture mode"=w215, "Handle in"=w220) -> ("error out"=w225:errorcluster, "Handle out"=w219:u32)  [unwired: 5 in, 2 out]
                n119 = call <userlib>:"tm_startcapture_40.vi"("error in (no error)"=w225, "Handle in"=w219) -> ("error out"=w224:errorcluster, "Handle out"=w228:u32)  [unwired: 8 in]
                n120 = call <userlib>:"tm_waitnextframe_40.vi"("error in (no error)"=w224, "Handle in"=w228) -> ("error out"=w223:errorcluster, "Frame Index"=w214:i32, "Handle out"=w218:u32)  [unwired: 6 in, 1 out]
                n121 = call <userlib>:"tm_getframe16_40.vi"("error in (no error)"=w223, "Frame Index"=w214, "Handle in"=w218) -> ("error out"=w222:errorcluster, "Handle out"=w217:u32)  [unwired: 5 in, 2 out]
                n122 = call <userlib>:"tm_stopcapture_40.vi"("error in (no error)"=w222, "Handle in"=w217) -> ("error out"=w221:errorcluster, "Handle out"=w216:u32)  [unwired: 8 in]
                n123 = call <userlib>:"tm_unpreparecapture_40.vi"("error in (no error)"=w221, "Handle in"=w216) -> ("error out"=w212:errorcluster, "Handle out"=w213:u32)  [unwired: 8 in]
                n124 = call <userlib>:"tm_closecamera_40.vi"("error in (no error)"=w212, "Handle in"=w213) -> ("error out"=w211:errorcluster)  [unwired: 9 in]
                n125 = call <userlib>:"tm_deinitialize_40.vi"("error in (no error)"=w211) -> ("error out"=w210:errorcluster)  [unwired: 10 in]
                n126 = local write "Error Cal"(w210) -> ()
              }
              frame #2 {
                n127 = global read "GlobalVariables.vi" "Toup Handle"() -> (w229:i32)
                n128 = dll-call lib="D:/amcamsdk.20210816/extras/labview/toupcam.dll" fn="Toupcam_Stop"("htoupcam"=w229) -> ("htoupcam"=w230:i32)  [unwired: 4 in, 2 out]
                n129 = dll-call lib="D:/amcamsdk.20210816/extras/labview/toupcam.dll" fn="Toupcam_Close"("htoupcam"=w230) -> ()  [unwired: 5 in, 2 out]
              }
              frame #3 {
                n130 = global read "GlobalVariables.vi" "Toup Temp Img"() -> (w232:T5)
                n131 = global read "GlobalVariables.vi" "Toup Ref Img"() -> (w231:T5)
                n132 = call "IMAQ Dispose"("Image"=w232) -> ()  [unwired: 5 in, 1 out]
                n133 = call "IMAQ Dispose"("Image"=w231) -> ()  [unwired: 5 in, 1 out]
              }
              frame #4 {
                n134 = Stop(stop? (T)=TRUE) -> ()
              }
            }
            n135 = global read "callback_Done.vi" "X Motor Reference"() -> (w205:refnum<k7>)
            n136 = global read "callback_Done.vi" "Y Motor Reference"() -> (w207:refnum<k7>)
            n137 = global read "callback_Done.vi" "Z Motor Reference"() -> (w206:refnum<k7>)
            n138 = invoke class="MG17Motor" method="StopCtrl"(reference=w205) -> ()  [unwired: 2 in, 3 out]
            n139 = invoke class="MG17Motor" method="StopCtrl"(reference=w207) -> ()  [unwired: 2 in, 3 out]
            n140 = invoke class="MG17Motor" method="StopCtrl"(reference=w206) -> ()  [unwired: 2 in, 3 out]
            n141 = local write "Stop"(FALSE) -> ()
          }
          frame 4 {
            w238 = u32 4215968 items=["SENSOR MODE"=4212128, "READOUT SPEED"=4211872, "READOUT DIRECTION"=4211904, "TRIGGER GLOBAL EXPOSURE"=2049680, "TRIGGER DELAY"=1066480, "INTERNAL TRIGGER HANDLING"=1066496, "SYNC READOUT SYSTEM BLANK"=1066528, "SENSOR TEMPERATURE"=2115232, "SENSOR COOLER STATUS"=2115280, "EXPOSURE TIME"=2049184, "DEFECT CORRECT MODE"=4670368, "BINNING"=4215968, "INTERNAL LINE SPEED"=4226000, "INTERNAL LINE INTERVAL"=4226016, "NUMBER OF OUTPUT TRIGGER CONNECTOR"=1852320, "OUTPUT TRIGGER SOURCE[0]"=1852576, "OUTPUT TRIGGER SOURCE[1]"=1852832, "OUTPUT TRIGGER SOURCE[2]"=1853088, "OUTPUT TRIGGER POLARITY[0]"=1852592, "OUTPUT TRIGGER POLARITY[1]"=1852848, "OUTPUT TRIGGER POLARITY[2]"=1853104, "OUTPUT TRIGGER ACTIVE[0]"=1852608, "OUTPUT TRIGGER ACTIVE[1]"=1852864, "OUTPUT TRIGGER ACTIVE[2]"=1853120, "OUTPUT TRIGGER DELAY[0]"=1852624, "OUTPUT TRIGGER DELAY[1]"=1852880, "OUTPUT TRIGGER DELAY[2]"=1853136, "OUTPUT TRIGGER PERIOD[0]"=1852640, "OUTPUT TRIGGER PERIOD[1]"=1852896, "OUTPUT TRIGGER PERIOD[2]"=1853152, "OUTPUT TRIGGER KIND[0]"=1852656, "OUTPUT TRIGGER KIND[1]"=1852912, "OUTPUT TRIGGER KIND[2]"=1853168, "OUTPUT TRIGGER BASE SENSOR[0]"=1852672, "OUTPUT TRIGGER BASE SENSOR[1]"=1852928, "OUTPUT TRIGGER BASE SENSOR[2]"=1853184, "OUTPUT TRIGGER PRE HSYNC COUNT"=1852704] ("Parameter")
            w246 = 0 items=["Snap", "Sequence"] ("Capture mode")
            w250 = u32 2049184 items=["SENSOR MODE"=4212128, "READOUT SPEED"=4211872, "READOUT DIRECTION"=4211904, "TRIGGER GLOBAL EXPOSURE"=2049680, "TRIGGER DELAY"=1066480, "INTERNAL TRIGGER HANDLING"=1066496, "SYNC READOUT SYSTEM BLANK"=1066528, "SENSOR TEMPERATURE"=2115232, "SENSOR COOLER STATUS"=2115280, "EXPOSURE TIME"=2049184, "DEFECT CORRECT MODE"=4670368, "BINNING"=4215968, "INTERNAL LINE SPEED"=4226000, "INTERNAL LINE INTERVAL"=4226016, "NUMBER OF OUTPUT TRIGGER CONNECTOR"=1852320, "OUTPUT TRIGGER SOURCE[0]"=1852576, "OUTPUT TRIGGER SOURCE[1]"=1852832, "OUTPUT TRIGGER SOURCE[2]"=1853088, "OUTPUT TRIGGER POLARITY[0]"=1852592, "OUTPUT TRIGGER POLARITY[1]"=1852848, "OUTPUT TRIGGER POLARITY[2]"=1853104, "OUTPUT TRIGGER ACTIVE[0]"=1852608, "OUTPUT TRIGGER ACTIVE[1]"=1852864, "OUTPUT TRIGGER ACTIVE[2]"=1853120, "OUTPUT TRIGGER DELAY[0]"=1852624, "OUTPUT TRIGGER DELAY[1]"=1852880, "OUTPUT TRIGGER DELAY[2]"=1853136, "OUTPUT TRIGGER PERIOD[0]"=1852640, "OUTPUT TRIGGER PERIOD[1]"=1852896, "OUTPUT TRIGGER PERIOD[2]"=1853152, "OUTPUT TRIGGER KIND[0]"=1852656, "OUTPUT TRIGGER KIND[1]"=1852912, "OUTPUT TRIGGER KIND[2]"=1853168, "OUTPUT TRIGGER BASE SENSOR[0]"=1852672, "OUTPUT TRIGGER BASE SENSOR[1]"=1852928, "OUTPUT TRIGGER BASE SENSOR[2]"=1853184, "OUTPUT TRIGGER PRE HSYNC COUNT"=1852704] ("Parameter")
            # "Calibration"
            n142 = call <userlib>:"tm_initialize_40.vi"() -> ("error out"=w254:errorcluster)  [unwired: 8 in, 3 out]
            n143 = call <userlib>:"tm_opencamera_40.vi"("error in (no error)"=w254) -> ("error out"=w253:errorcluster, "Handle out"=w252:u32)  [unwired: 8 in, 1 out]
            n144 = local read "Binning"() -> (w237:dbl)
            n145 = call <userlib>:"tm_setarea_40.vi"("error in (no error)"=w253, "Sub Region"=w251, "Handle in"=w252) -> ("error out"=w239:errorcluster, "Handle out"=w242:u32)  [unwired: 7 in]
            n146 = call <userlib>:"tm_setparameter_40.vi"("error in (no error)"=w239, "Value in"=w237, "Parameter"=w238, "Handle in"=w242) -> ("error out"=w240:errorcluster, "Handle out"=w241:u32)  [unwired: 6 in]
            n147 = call <userlib>:"tm_setparameter_40.vi"("error in (no error)"=w240, "Value in"=w249, "Parameter"=w250, "Handle in"=w241) -> ("error out"=w248:errorcluster, "Handle out"=w247:u32)  [unwired: 6 in]
            n148 = call <userlib>:"tm_preparecapture_40.vi"("error in (no error)"=w248, "Capture mode"=w246, "Handle in"=w247) -> ("error out"=w244:errorcluster, "Handle out"=w245:u32)  [unwired: 5 in, 2 out]
            n149 = stacked-sequence {
              tunnel: "Z count" -> [_ w290 _]
              tunnel: "Y count" -> [_ w289 _]
              tunnel: "X count" -> [_ w288 _]
              tunnel: w245 -> [_ w287 _]
              tunnel: w244 -> [_ w286 _]
              tunnel: w249 -> [w270 _ _]
              tunnel: w251 -> [w269 _ _]
              tunnel: "LED Power" -> [w268 _ _]
              tunnel: "CalRepeat" -> [w257 w285 _]
              frame #0 {
                # "Initiaize calibration sequence"
                n150 = local read "Toup Crop 5440x3648"() -> (w265:T2)
                n151 = local read "ExpoGain"() -> (w263:u16)
                n152 = local write "Calibrating..."(TRUE ("Calibrating...")) -> ()
                n153 = call <vilib>:"Check if File or Folder Exists.vi"("path"="Calibration Folder") -> ("file or folder exists?"=w278:bool, "dup path"=w279:path)  [unwired: 8 in, 1 out]
                n154 = Cluster To Array(cluster=w269) -> (array=w266:i32[])
                n155 = local read "Binning"() -> (w262:dbl)
                n156 = case shown="False" w278 {
                  tunnel: w279 -> [w283 w284]
                  tunnel: [w282 w284] -> w277
                  frame False {
                    n157 = Create Folder(path (use dialog)=w283) -> (created path=w282:path)  [unwired: 2 in, 2 out]
                  }
                  frame True {
                  }
                }
                n158 = local read "CalWait (ms)"() -> (w256:dbl)
                n159 = local read "Expotime (ms)"() -> (w267:dbl)
                n160 = local read "Z init"() -> (w258:dbl)
                n161 = local read "X count"() -> (w276:i32)
                n162 = local read "Y count"() -> (w275:i32)
                n163 = local read "Z count"() -> (w274:i32)
                n164 = local read "X init"() -> (w260:dbl)
                n165 = local read "Y init"() -> (w259:dbl)
                n166 = local read "X size"() -> (w273:dbl)
                n167 = local read "Y size"() -> (w272:dbl)
                n168 = local read "Z size"() -> (w271:dbl)
                n169 = Cluster To Array(cluster=w265) -> (array=w264:i32[])
                n170 = script code="saveCalibrationMetafile;"("path"=w277, "xCount"=w276, "yCount"=w275, "zCount"=w274, "xStep"=w273, "yStep"=w272, "zStep"=w271, "orcaExp"=w270, "LEDPower"=w268, "AmExp"=w267, "OrcaCrop"=w266, "AmCrop"=w264, "AmGain"=w263, "binning"=w262, "Xinit"=w260, "Yinit"=w259, "Zinit"=w258, "CalRepeat"=w257, "CalWait"=w256) -> ()  [unwired: 1 in, 1 out]
                "Cal Count" <- 0.0 ("Count")
              }
              frame #1 {
                # "Calibration sequence"
                n171 = for {
                  N: w285 -> [_]
                  tunnel: w290 -> [w301]
                  tunnel: w289 -> [w300]
                  tunnel: w288 -> [w299]
                  tunnel: w287 -> [w298]
                  tunnel: w286 -> [w297]
                  i -> [w296]
                  n172 = flat-sequence {
                    tunnel: w297 -> [w303]
                    tunnel: w298 -> [w304]
                    tunnel: w299 -> [w305]
                    tunnel: w300 -> [w306]
                    tunnel: w301 -> [w307]
                    tunnel: [w307] -> w295
                    tunnel: [w306] -> w294
                    tunnel: [w305] -> w293
                    tunnel: [w304] -> w292
                    tunnel: [w303] -> w291
                    tunnel: w296 -> [w308]
                    tunnel: w295 -> [w313]
                    tunnel: w294 -> [w312]
                    tunnel: w293 -> [w311]
                    tunnel: w292 -> [w310]
                    tunnel: w291 -> [w309]
                    frame #0 {
                      n173 = call <userlib>:"U3 eDAC Example.vi"("Voltage"=5.0) -> ()  [unwired: 10 in, 1 out]
                    }
                    frame #1 {
                      n174 = for {
                        N: w311 -> [_]
                        tunnel: w313 -> [w318]
                        tunnel: w312 -> [w317]
                        tunnel: w310 -> [w316]
                        tunnel: w309 -> [w315]
                        tunnel: w308 -> [w314]
                        i -> [w320]
                        stop <- w319 stop-if-true
                        n175 = for {
                          N: w317 -> [_]
                          tunnel: w320 -> [w326]
                          tunnel: [w325] -> w319
                          tunnel: w318 -> [w324]
                          tunnel: w316 -> [w323]
                          tunnel: w315 -> [w322]
                          tunnel: w314 -> [w321]
                          i -> [w327]
                          stop <- w325 stop-if-true
                          n176 = for {
                            N: w324 -> [_]
                            tunnel: w327 -> [w331]
                            tunnel: w326 -> [w333]
                            tunnel: [w332] -> w325
                            tunnel: w323 -> [w329]
                            tunnel: w322 -> [w330]
                            tunnel: w321 -> [w328]
                            i -> [w334]
                            stop <- w332 stop-if-true
                            n177 = stacked-sequence {
                              tunnel: w334 -> [_ _ _ w370 _ _ w403 _]
                              tunnel: w331 -> [_ _ w358 _ _ _ w420 _]
                              tunnel: [_ _ _ _ _ _ _ "Abort"] -> w332
                              tunnel: w333 -> [_ w345 _ _ _ _ w402 _]
                              tunnel: w330 -> [_ _ _ _ _ w387 w408 _]
                              tunnel: w329 -> [_ _ _ _ _ w388 w415 w427]
                              tunnel: w328 -> [_ _ _ _ _ _ w404 _]
                              frame #0 {
                                n178 = case shown="True" "Z Retreat" {
                                frame False {
                                }
                                frame True {
                                n179 = flat-sequence {
                                frame #0 {
                                n180 = global read "callback_Done.vi" "Z Motor Reference"() -> (w339:refnum<k7>)
                                n181 = invoke class="MG17Motor" method="MoveAbsoluteEnc"(reference=w339, "lChanID"=0, "fAbsPosCh1"="Z Retreat Pos", "fAbsPosCh2"="Z Retreat Pos", "lTimeInc"=1000, "bWait"=FALSE) -> ("fAbsPosCh1"=w337:sgl)  [unwired: 2 in, 7 out]
                                n182 = global write "callback_Done.vi" "Z Motor done"(FALSE ("Motor done")) -> ()
                                n183 = local write "Z Pos (mm)"(w337) -> ()
                                }
                                frame #1 {
                                n184 = while {
                                stop <- w344 stop-if-true
                                n185 = global read "callback_Done.vi" "Z Motor done"() -> (w344:bool)
                                }
                                n186 = Wait (ms)(milliseconds to wait=100) -> ()  [unwired: 1 out]
                                }
                                }
                                }
                                }
                              }
                              frame #1 {
                                # "Change x axis location of point source"
                                n187 = global read "callback_Done.vi" "X Motor Reference"() -> (w348:refnum<k7>)
                                n188 = Multiply(x="X size", y=w345) -> (x*y=w356:dbl)
                                n189 = Add(x=w356, y="X init") -> (x+y=w349:dbl)
                                n190 = invoke class="MG17Motor" method="MoveAbsoluteEnc"(reference=w348, "lChanID"=0, "fAbsPosCh1"=w349, "fAbsPosCh2"=w349, "lTimeInc"=1000, "bWait"=FALSE) -> ("fAbsPosCh1"=→"X Pos (mm)":sgl)  [unwired: 2 in, 7 out]
                                n191 = global write "callback_Done.vi" "X Motor done"(FALSE ("Motor done")) -> ()
                                n192 = Wait (ms)(milliseconds to wait=0) -> ()  [unwired: 1 out]
                                "Moving..." <- TRUE ("Waiting...")
                              }
                              frame #2 {
                                # "Change y axis location of point source"
                                n193 = Multiply(x="Y size", y=w358) -> (x*y=w367:dbl)
                                n194 = global read "callback_Done.vi" "Y Motor Reference"() -> (w362:refnum<k7>)
                                n195 = Add(x=w367, y="Y init") -> (x+y=w361:dbl)
                                n196 = Wait (ms)(milliseconds to wait=0) -> ()  [unwired: 1 out]
                                n197 = invoke class="MG17Motor" method="MoveAbsoluteEnc"(reference=w362, "lChanID"=0, "fAbsPosCh1"=w361, "fAbsPosCh2"=w361, "lTimeInc"=1000, "bWait"=FALSE) -> ("fAbsPosCh1"=→"Y Pos (mm)":sgl)  [unwired: 2 in, 7 out]
                                n198 = global write "callback_Done.vi" "Y Motor done"(FALSE ("Motor done")) -> ()
                              }
                              frame #3 {
                                # "Change z axis location of point source, if needed"
                                n199 = global read "callback_Done.vi" "Z Motor Reference"() -> (w374:refnum<k7>)
                                n200 = Multiply(x="Z size", y=w370) -> (x*y=w379:dbl)
                                n201 = Add(x=w379, y="Z init") -> (x+y=w373:dbl)
                                n202 = invoke class="MG17Motor" method="MoveAbsoluteEnc"(reference=w374, "lChanID"=0, "fAbsPosCh1"=w373, "fAbsPosCh2"=w373, "lTimeInc"=1000, "bWait"=FALSE) -> ("fAbsPosCh1"=→"Z Pos (mm)":sgl)  [unwired: 2 in, 7 out]
                                n203 = global write "callback_Done.vi" "Z Motor done"(FALSE ("Motor done")) -> ()
                              }
                              frame #4 {
                                # "(If moving) Wait until X,Y,Z motion is finished."
                                n204 = while {
                                stop <- w382 stop-if-true
                                n205 = global read "callback_Done.vi" "Z Motor done"() -> (w386:bool)
                                n206 = global read "callback_Done.vi" "Y Motor done"() -> (w384:bool)
                                n207 = global read "callback_Done.vi" "X Motor done"() -> (w383:bool)
                                n208 = And(x=w384, y=w383) -> (x .and. y?=w385:bool)
                                n209 = And(x=w386, y=w385) -> (x .and. y?=w382:bool)
                                }
                                n210 = Wait (ms)(milliseconds to wait=100) -> ()  [unwired: 1 out]
                              }
                              frame #5 {
                                # "Throw one frame out"
                                n211 = flat-sequence {
                                tunnel: w388 -> [w395]
                                tunnel: w387 -> [w390]
                                frame #0 {
                                n212 = call <userlib>:"tm_startcapture_40.vi"("error in (no error)"=w390, "Handle in"=w395) -> ("error out"=w391:errorcluster, "Handle out"=w394:u32)  [unwired: 8 in]
                                n213 = call <userlib>:"tm_waitnextframe_40.vi"("error in (no error)"=w391, "Handle in"=w394) -> ("error out"=w397:errorcluster, "Frame Index"=w396:i32, "Handle out"=w398:u32)  [unwired: 6 in, 1 out]
                                n214 = call <userlib>:"tm_getframe16_40.vi"("error in (no error)"=w397, "Frame Index"=w396, "Handle in"=w398) -> ("error out"=w392:errorcluster, "Handle out"=w393:u32)  [unwired: 5 in, 2 out]
                                n215 = call <userlib>:"tm_stopcapture_40.vi"("error in (no error)"=w392, "Handle in"=w393) -> ("error out"=w389:errorcluster)  [unwired: 8 in, 1 out]
                                n216 = local write "Error Cal"(w389) -> ()
                                }
                                frame #1 {
                                n217 = local read "Wait (ms)"() -> (w399:dbl)
                                n218 = Wait (ms)(milliseconds to wait=w399) -> ()  [unwired: 1 out]
                                }
                                frame #2 {
                                n219 = disable-structure shown="Disabled" {
                                frame Disabled {
                                n220 = call <userlib>:"U3 eDAC Example.vi"("Voltage"=5.0) -> ()  [unwired: 10 in, 1 out]
                                }
                                frame Enabled {
                                }
                                }
                                }
                                frame #3 {
                                n221 = disable-structure shown="Disabled" {
                                frame Disabled {
                                n222 = Wait (ms)(milliseconds to wait=u32 1000) -> ()  [unwired: 1 out]
                                }
                                frame Enabled {
                                }
                                }
                                }
                                }
                              }
                              frame #6 {
                                w417 = T6 1 items=["no dialog", "OK message", "continue or stop message", "OK message + warnings", "continue/stop + warnings"] ("type of dialog (OK msg:1)")
                                # "Capture and save HDR image"
                                n223 = call <userlib>:"tm_startcapture_40.vi"("error in (no error)"=w408, "Handle in"=w415) -> ("error out"=w409:errorcluster, "Handle out"=w414:u32)  [unwired: 8 in]
                                n224 = call <userlib>:"tm_waitnextframe_40.vi"("error in (no error)"=w409, "Handle in"=w414) -> ("error out"=w410:errorcluster, "Frame Index"=w407:i32, "Handle out"=w413:u32)  [unwired: 6 in, 1 out]
                                n225 = local write "Moving..."(FALSE ("Waiting...")) -> ()
                                n226 = Format Into String(format string="x%d_y%d_z%d_t%d", w402, w420, w403, w404) -> (resulting string=w419:string)  [unwired: 2 in, 1 out]
                                n227 = call <userlib>:"tm_getframe16_40.vi"("error in (no error)"=w410, "Frame Index"=w407, "Handle in"=w413) -> ("error out"=w411:errorcluster, "Data"=w406:u16[][], "Handle out"=w412:u32)  [unwired: 5 in, 1 out]
                                n228 = property on="objRef" class="IntGraph (strict)"() -> ("Value"=w416:u8[][])  [unwired: 2 in, 2 out]
                                n229 = local write "Image"(w406) -> ()
                                n230 = call <userlib>:"tm_stopcapture_40.vi"("error in (no error)"=w411, "Handle in"=w412) -> ("error out"=w405:errorcluster)  [unwired: 8 in, 1 out]
                                n231 = script code="%imgHDR = single(imgHDR);\n%objRef = single(objRef);\nsave([path,'/',name],'objCCM','objRef','xPos','yPos','zPos');"("name"=w419, "objRef"=w416, "objCCM"=w406) -> ("??"=w418:errorcluster)  [unwired: 1 in]
                                n232 = local write "Error Cal"(w405) -> ()
                                n233 = call <vilib>:"Simple Error Handler.vi"("type of dialog (OK msg:1)"=w417, "error in (no error)"=w418) -> ()  [unwired: 3 in, 5 out]
                                "Saving..." <- TRUE ("Acquiring...")
                              }
                              frame #7 {
                                # "Loop rate counter"
                                # "Calculate calibration frame rate and display."
                                n234 = local write "Saving..."(FALSE ("Saving...")) -> ()
                                n235 = local read "Cal Count"() -> (w425:dbl)
                                n236 = case shown="True" "Abort" {
                                tunnel: w427 -> [_ w434]
                                frame False {
                                }
                                frame True {
                                n237 = call <userlib>:"tm_unpreparecapture_40.vi"("Handle in"=w434) -> ("error out"=w433:errorcluster, "Handle out"=w432:u32)  [unwired: 9 in]
                                n238 = local write "Calibrating..."(FALSE) -> ()
                                n239 = call <userlib>:"tm_closecamera_40.vi"("error in (no error)"=w433, "Handle in"=w432) -> ("error out"=w431:errorcluster)  [unwired: 9 in]
                                n240 = call <userlib>:"tm_deinitialize_40.vi"("error in (no error)"=w431) -> ()  [unwired: 10 in, 1 out]
                                }
                                }
                                n241 = Increment(x=w425) -> (x+1=w424:dbl)
                                n242 = local write "Cal Count"(w424) -> ()
                                n243 = disable-structure shown="Disabled" {
                                frame Disabled {
                                n244 = call <userlib>:"U3 eDAC Example.vi"("Voltage"=0.0) -> ()  [unwired: 10 in, 1 out]
                                }
                                frame Enabled {
                                }
                                }
                              }
                            }
                          }
                        }
                      }
                    }
                    frame #2 {
                      n245 = call <userlib>:"U3 eDAC Example.vi"("Voltage"=0.0) -> ()  [unwired: 10 in, 1 out]
                    }
                    frame #3 {
                      n246 = Wait (ms)(milliseconds to wait="CalWait (ms)") -> ()  [unwired: 1 out]
                    }
                  }
                }
              }
              frame #2 {
                w438 = u16 6 items=["Wait", "Acquire Live", "Acquire Single", "Terminate", "Calibration", "Macro", "Wait Prep"] ("Imaging status")
                # "Wrap up the calibration"
                n247 = local write "Abort"(FALSE ("Abort")) -> ()
                n248 = local write "Calibrating..."(FALSE ("Calibrating...")) -> ()
                n249 = local write "Imaging status"(w438) -> ()
                n250 = call <userlib>:"U3 eDAC Example.vi"("Voltage"=0.0) -> ()  [unwired: 10 in, 1 out]
              }
            }
          }
          frame 5 {
            w442 = u32 4215968 items=["SENSOR MODE"=4212128, "READOUT SPEED"=4211872, "READOUT DIRECTION"=4211904, "TRIGGER GLOBAL EXPOSURE"=2049680, "TRIGGER DELAY"=1066480, "INTERNAL TRIGGER HANDLING"=1066496, "SYNC READOUT SYSTEM BLANK"=1066528, "SENSOR TEMPERATURE"=2115232, "SENSOR COOLER STATUS"=2115280, "EXPOSURE TIME"=2049184, "DEFECT CORRECT MODE"=4670368, "BINNING"=4215968, "INTERNAL LINE SPEED"=4226000, "INTERNAL LINE INTERVAL"=4226016, "NUMBER OF OUTPUT TRIGGER CONNECTOR"=1852320, "OUTPUT TRIGGER SOURCE[0]"=1852576, "OUTPUT TRIGGER SOURCE[1]"=1852832, "OUTPUT TRIGGER SOURCE[2]"=1853088, "OUTPUT TRIGGER POLARITY[0]"=1852592, "OUTPUT TRIGGER POLARITY[1]"=1852848, "OUTPUT TRIGGER POLARITY[2]"=1853104, "OUTPUT TRIGGER ACTIVE[0]"=1852608, "OUTPUT TRIGGER ACTIVE[1]"=1852864, "OUTPUT TRIGGER ACTIVE[2]"=1853120, "OUTPUT TRIGGER DELAY[0]"=1852624, "OUTPUT TRIGGER DELAY[1]"=1852880, "OUTPUT TRIGGER DELAY[2]"=1853136, "OUTPUT TRIGGER PERIOD[0]"=1852640, "OUTPUT TRIGGER PERIOD[1]"=1852896, "OUTPUT TRIGGER PERIOD[2]"=1853152, "OUTPUT TRIGGER KIND[0]"=1852656, "OUTPUT TRIGGER KIND[1]"=1852912, "OUTPUT TRIGGER KIND[2]"=1853168, "OUTPUT TRIGGER BASE SENSOR[0]"=1852672, "OUTPUT TRIGGER BASE SENSOR[1]"=1852928, "OUTPUT TRIGGER BASE SENSOR[2]"=1853184, "OUTPUT TRIGGER PRE HSYNC COUNT"=1852704] ("Parameter")
            w451 = 0 items=["Snap", "Sequence"] ("Capture mode")
            w454 = u32 2049184 items=["SENSOR MODE"=4212128, "READOUT SPEED"=4211872, "READOUT DIRECTION"=4211904, "TRIGGER GLOBAL EXPOSURE"=2049680, "TRIGGER DELAY"=1066480, "INTERNAL TRIGGER HANDLING"=1066496, "SYNC READOUT SYSTEM BLANK"=1066528, "SENSOR TEMPERATURE"=2115232, "SENSOR COOLER STATUS"=2115280, "EXPOSURE TIME"=2049184, "DEFECT CORRECT MODE"=4670368, "BINNING"=4215968, "INTERNAL LINE SPEED"=4226000, "INTERNAL LINE INTERVAL"=4226016, "NUMBER OF OUTPUT TRIGGER CONNECTOR"=1852320, "OUTPUT TRIGGER SOURCE[0]"=1852576, "OUTPUT TRIGGER SOURCE[1]"=1852832, "OUTPUT TRIGGER SOURCE[2]"=1853088, "OUTPUT TRIGGER POLARITY[0]"=1852592, "OUTPUT TRIGGER POLARITY[1]"=1852848, "OUTPUT TRIGGER POLARITY[2]"=1853104, "OUTPUT TRIGGER ACTIVE[0]"=1852608, "OUTPUT TRIGGER ACTIVE[1]"=1852864, "OUTPUT TRIGGER ACTIVE[2]"=1853120, "OUTPUT TRIGGER DELAY[0]"=1852624, "OUTPUT TRIGGER DELAY[1]"=1852880, "OUTPUT TRIGGER DELAY[2]"=1853136, "OUTPUT TRIGGER PERIOD[0]"=1852640, "OUTPUT TRIGGER PERIOD[1]"=1852896, "OUTPUT TRIGGER PERIOD[2]"=1853152, "OUTPUT TRIGGER KIND[0]"=1852656, "OUTPUT TRIGGER KIND[1]"=1852912, "OUTPUT TRIGGER KIND[2]"=1853168, "OUTPUT TRIGGER BASE SENSOR[0]"=1852672, "OUTPUT TRIGGER BASE SENSOR[1]"=1852928, "OUTPUT TRIGGER BASE SENSOR[2]"=1853184, "OUTPUT TRIGGER PRE HSYNC COUNT"=1852704] ("Parameter")
            # "Support Surface"
            n251 = call <userlib>:"tm_initialize_40.vi"() -> ("error out"=w457:errorcluster)  [unwired: 8 in, 3 out]
            n252 = call <userlib>:"tm_opencamera_40.vi"("error in (no error)"=w457) -> ("error out"=w456:errorcluster, "Handle out"=w455:u32)  [unwired: 8 in, 1 out]
            n253 = call <userlib>:"tm_setarea_40.vi"("error in (no error)"=w456, "Sub Region"=w448, "Handle in"=w455) -> ("error out"=w444:errorcluster, "Handle out"=w446:u32)  [unwired: 7 in]
            n254 = call <userlib>:"tm_setparameter_40.vi"("error in (no error)"=w444, "Value in"="Binning", "Parameter"=w442, "Handle in"=w446) -> ("error out"=w443:errorcluster, "Handle out"=w445:u32)  [unwired: 6 in]
            n255 = call <userlib>:"tm_setparameter_40.vi"("error in (no error)"=w443, "Value in"=w447, "Parameter"=w454, "Handle in"=w445) -> ("error out"=w453:errorcluster, "Handle out"=w452:u32)  [unwired: 6 in]
            n256 = call <userlib>:"tm_preparecapture_40.vi"("error in (no error)"=w453, "Capture mode"=w451, "Handle in"=w452) -> ("error out"=w449:errorcluster, "Handle out"=w450:u32)  [unwired: 5 in, 2 out]
            n257 = stacked-sequence {
              tunnel: w450 -> [_ w484 _]
              tunnel: w449 -> [_ w483 _]
              tunnel: w447 -> [w472 _ _]
              tunnel: w448 -> [w471 _ _]
              frame #0 {
                # "Initiaize calibration sequence"
                n258 = local read "Toup Crop 5440x3648"() -> (w461:T2)
                n259 = script code="Surface = genSurface2(Support);\nSurface(:, 1:20) = [];\nz = [-0.01, -0.005, 0, 0.005, 0.01];\nSurface = genZstack(Surface, z);\nlenSurface = length(Surface);"() -> ("lenSurface"=→"lenSurface":dbl, "Support"=w468:dbl[][], "Surface"=w467:dbl[][])  [unwired: 1 in, 1 out]
                n260 = local read "Calibration Folder"() -> (w470:path)
                n261 = local read "LED Power"() -> (w466:dbl)
                n262 = Get Date/Time In Seconds() -> (seconds since 1Jan1904=→"Start Time":timestamp)
                n263 = local write "Calibrating... 2"(TRUE ("Calibrating...")) -> ()
                n264 = call <vilib>:"Check if File or Folder Exists.vi"("path"=w470) -> ("file or folder exists?"=w474:bool, "dup path"=w475:path)  [unwired: 8 in, 1 out]
                n265 = Cluster To Array(cluster=w471) -> (array=w462:i32[])
                n266 = case shown="False" w474 {
                  tunnel: w475 -> [w478 w479]
                  tunnel: [w477 w479] -> w473
                  frame False {
                    n267 = Create Folder(path (use dialog)=w478) -> (created path=w477:path)  [unwired: 2 in, 2 out]
                  }
                  frame True {
                  }
                }
                n268 = local read "Binning"() -> (w459:dbl)
                n269 = local read "ExpoGain"() -> (w463:u16)
                n270 = local read "Expotime (ms)"() -> (w465:dbl)
                n271 = local read "FrameAve"() -> (w464:dbl)
                n272 = Cluster To Array(cluster=w461) -> (array=w460:i32[])
                n273 = script code="saveSupportMetafile;"("path"=w473, "Support"=w468, "orcaExp"=w472, "Surface"=w467, "LEDPower"=w466, "AmExp"=w465, "FrameAve"=w464, "AmGain"=w463, "OrcaCrop"=w462, "AmCrop"=w460, "binning"=w459) -> ()  [unwired: 1 in, 1 out]
              }
              frame #1 {
                # "Calibration sequence"
                n274 = local read "lenSurface"() -> (w482:dbl)
                n275 = Subtract(x=w482, y=1.0) -> (x-y=w480:dbl)
                n276 = for {
                  N: w480 -> [_]
                  tunnel: w484 -> [w489]
                  tunnel: w483 -> [w488]
                  i -> [w487]
                  stop <- w490 stop-if-true
                  n277 = Add(x=1, y=w487) -> (x+y=w485:i32)
                  "Count" <- w485
                  n278 = stacked-sequence {
                    tunnel: [_ _ _ _ _ _ "Abort 2"] -> w490
                    tunnel: w485 -> [w492 w508 w519 _ _ w540 _]
                    tunnel: w488 -> [_ _ _ _ w526 w541 _]
                    tunnel: w489 -> [_ _ _ _ w527 w542 w570]
                    frame #0 {
                      # "Change x axis location of point source"
                      n279 = script code="xPos = Surface(1,i);"("i"=w492) -> ("xPos"=w491:dbl)  [unwired: 1 in, 1 out]
                      n280 = global read "callback_Done.vi" "X Motor Reference"() -> (w495:refnum<k7>)
                      n281 = invoke class="MG17Motor" method="MoveAbsoluteEnc"(reference=w495, "lChanID"=0, "fAbsPosCh1"=w491, "fAbsPosCh2"=w491, "lTimeInc"=1000, "bWait"=FALSE) -> ("fAbsPosCh1"=→"X Pos (mm) 2":sgl)  [unwired: 2 in, 7 out]
                      n282 = global write "callback_Done.vi" "X Motor done"(FALSE ("Motor done")) -> ()
                      n283 = Wait (ms)(milliseconds to wait=0) -> ()  [unwired: 1 out]
                      "Moving... 2" <- TRUE ("Waiting...")
                    }
                    frame #1 {
                      # "Change y axis location of point source"
                      n284 = script code="yPos = Surface(2,i);"("i"=w508) -> ("yPos"=w507:dbl)  [unwired: 1 in, 1 out]
                      n285 = global read "callback_Done.vi" "Y Motor Reference"() -> (w503:refnum<k7>)
                      n286 = Wait (ms)(milliseconds to wait=0) -> ()  [unwired: 1 out]
                      n287 = invoke class="MG17Motor" method="MoveAbsoluteEnc"(reference=w503, "lChanID"=0, "fAbsPosCh1"=w507, "fAbsPosCh2"=w507, "lTimeInc"=1000, "bWait"=FALSE) -> ("fAbsPosCh1"=→"Y Pos (mm) 2":sgl)  [unwired: 2 in, 7 out]
                      n288 = global write "callback_Done.vi" "Y Motor done"(FALSE ("Motor done")) -> ()
                    }
                    frame #2 {
                      # "Change z axis location of point source, if needed"
                      n289 = script code="zPos = Surface(3,i);"("i"=w519) -> ("zPos"=w512:dbl)  [unwired: 1 in, 1 out]
                      n290 = Add(x="Shrink", y=w512) -> (x+y=w510:dbl)
                      n291 = global read "callback_Done.vi" "Z Motor Reference"() -> (w515:refnum<k7>)
                      n292 = invoke class="MG17Motor" method="MoveAbsoluteEnc"(reference=w515, "lChanID"=0, "fAbsPosCh1"=w510, "fAbsPosCh2"=w510, "lTimeInc"=1000, "bWait"=FALSE) -> ("fAbsPosCh1"=→"Z Pos (mm) 2":sgl)  [unwired: 2 in, 7 out]
                      n293 = global write "callback_Done.vi" "Z Motor done"(FALSE ("Motor done")) -> ()
                    }
                    frame #3 {
                      # "(If moving) Wait until X,Y,Z motion is finished."
                      n294 = while {
                        stop <- w521 stop-if-true
                        n295 = global read "callback_Done.vi" "Z Motor done"() -> (w525:bool)
                        n296 = global read "callback_Done.vi" "Y Motor done"() -> (w523:bool)
                        n297 = global read "callback_Done.vi" "X Motor done"() -> (w522:bool)
                        n298 = And(x=w523, y=w522) -> (x .and. y?=w524:bool)
                        n299 = And(x=w525, y=w524) -> (x .and. y?=w521:bool)
                      }
                      n300 = Wait (ms)(milliseconds to wait=100) -> ()  [unwired: 1 out]
                    }
                    frame #4 {
                      # "Throw one frame out"
                      n301 = flat-sequence {
                        tunnel: w527 -> [w534]
                        tunnel: w526 -> [w529]
                        frame #0 {
                          n302 = call <userlib>:"tm_startcapture_40.vi"("error in (no error)"=w529, "Handle in"=w534) -> ("error out"=w530:errorcluster, "Handle out"=w533:u32)  [unwired: 8 in]
                          n303 = call <userlib>:"tm_waitnextframe_40.vi"("error in (no error)"=w530, "Handle in"=w533) -> ("error out"=w536:errorcluster, "Frame Index"=w535:i32, "Handle out"=w537:u32)  [unwired: 6 in, 1 out]
                          n304 = call <userlib>:"tm_getframe16_40.vi"("error in (no error)"=w536, "Frame Index"=w535, "Handle in"=w537) -> ("error out"=w531:errorcluster, "Handle out"=w532:u32)  [unwired: 5 in, 2 out]
                          n305 = call <userlib>:"tm_stopcapture_40.vi"("error in (no error)"=w531, "Handle in"=w532) -> ("error out"=w528:errorcluster)  [unwired: 8 in, 1 out]
                          n306 = local write "Error Surf"(w528) -> ()
                        }
                        frame #1 {
                          n307 = local read "Wait (ms) 2"() -> (w538:dbl)
                          n308 = Wait (ms)(milliseconds to wait=w538) -> ()  [unwired: 1 out]
                        }
                      }
                    }
                    frame #5 {
                      # "Capture and save HDR image"
                      n309 = for {
                        N: "FrameAve" -> [_]
                        tunnel: w542 -> [w562]
                        tunnel: w541 -> [w555]
                        tunnel: w540 -> [w550]
                        tunnel: "FrameAve" -> [w547]
                        i -> [w549]
                        w563 = T6 1 items=["no dialog", "OK message", "continue or stop message", "OK message + warnings", "continue/stop + warnings"] ("type of dialog (OK msg:1)")
                        n310 = call <userlib>:"tm_startcapture_40.vi"("error in (no error)"=w555, "Handle in"=w562) -> ("error out"=w556:errorcluster, "Handle out"=w561:u32)  [unwired: 8 in]
                        n311 = property on="objRef" class="IntGraph (strict)"() -> ("Value"=w551:u8[][])  [unwired: 2 in, 2 out]
                        n312 = call <userlib>:"tm_waitnextframe_40.vi"("error in (no error)"=w556, "Handle in"=w561) -> ("error out"=w557:errorcluster, "Frame Index"=w554:i32, "Handle out"=w560:u32)  [unwired: 6 in, 1 out]
                        n313 = local write "Moving... 2"(FALSE ("Waiting...")) -> ()
                        n314 = local read "Orca Exposure"() -> (w545:dbl)
                        n315 = Format Into String(format string="%d", w550) -> (resulting string=w565:string)  [unwired: 2 in, 1 out]
                        n316 = local read "Expotime (ms)"() -> (w546:dbl)
                        n317 = call <userlib>:"tm_getframe16_40.vi"("error in (no error)"=w557, "Frame Index"=w554, "Handle in"=w560) -> ("error out"=w558:errorcluster, "Data"=w553:u16[][], "Handle out"=w559:u32)  [unwired: 5 in, 1 out]
                        n318 = local write "Image"(w553) -> ()
                        n319 = call <userlib>:"tm_stopcapture_40.vi"("error in (no error)"=w558, "Handle in"=w559) -> ("error out"=w552:errorcluster)  [unwired: 8 in, 1 out]
                        n320 = local write "Error Surf"(w552) -> ()
                        n321 = script code="Frame = num2str(Frame);\nUnderscore = '_';\nif FrameAve == 1\nname = [CapPos];\nelse\nname = [CapPos Underscore Frame];\nend\nsave([path,'/',name],'objCCM','objRef','xPos','yPos','zPos');\n\n\n% [AmExp, OrcaExp] = autoExposure(objCCM, objRef, AmExp, OrcaExp);"("CapPos"=w565, "objRef"=w551, "objCCM"=w553, "Frame"=w549, "FrameAve"=w547, "AmExp"=w546, "OrcaExp"=w545) -> ("??"=w564:errorcluster, "OrcaExp"=w543:dbl, "AmExp"=w544:dbl)  [unwired: 1 in]
                        n322 = Wait (ms)(milliseconds to wait=u32 200) -> ()  [unwired: 1 out]
                        n323 = call <vilib>:"Simple Error Handler.vi"("type of dialog (OK msg:1)"=w563, "error in (no error)"=w564) -> ()  [unwired: 3 in, 5 out]
                        n324 = local write "Orca Exposure"(w543) -> ()
                        n325 = local write "Expotime (ms)"(w544) -> ()
                        "Saving... 2" <- TRUE ("Acquiring...")
                      }
                    }
                    frame #6 {
                      # "Loop rate counter"
                      # "Calculate calibration frame rate and display."
                      n326 = flat-sequence {
                        frame #0 {
                        }
                        frame #1 {
                        }
                      }
                      n327 = local write "Saving... 2"(FALSE ("Saving...")) -> ()
                      n328 = case shown="False" "Abort 2" {
                        tunnel: w570 -> [_ w575]
                        frame False {
                        }
                        frame True {
                          n329 = call <userlib>:"tm_unpreparecapture_40.vi"("Handle in"=w575) -> ("error out"=w574:errorcluster, "Handle out"=w573:u32)  [unwired: 9 in]
                          n330 = call <userlib>:"tm_closecamera_40.vi"("error in (no error)"=w574, "Handle in"=w573) -> ("error out"=w572:errorcluster)  [unwired: 9 in]
                          n331 = call <userlib>:"tm_deinitialize_40.vi"("error in (no error)"=w572) -> ()  [unwired: 10 in, 1 out]
                        }
                      }
                    }
                  }
                }
              }
              frame #2 {
                w578 = u16 6 items=["Wait", "Acquire Live", "Acquire Single", "Terminate", "Calibration", "Macro", "Wait Prep"] ("Imaging status")
                # "Wrap up the calibration"
                n332 = local write "Calibrating... 2"(FALSE ("Calibrating...")) -> ()
                n333 = local write "Abort 2"(FALSE ("Abort")) -> ()
                n334 = local write "Generate Surface & Go"(FALSE) -> ()
                n335 = local write "Imaging status"(w578) -> ()
                n336 = call <userlib>:"U3 eDAC Example.vi"("Voltage"=0.0) -> ()  [unwired: 10 in, 1 out]
              }
            }
          }
          frame 7 {
            w582 = u32 4215968 items=["SENSOR MODE"=4212128, "READOUT SPEED"=4211872, "READOUT DIRECTION"=4211904, "TRIGGER GLOBAL EXPOSURE"=2049680, "TRIGGER DELAY"=1066480, "INTERNAL TRIGGER HANDLING"=1066496, "SYNC READOUT SYSTEM BLANK"=1066528, "SENSOR TEMPERATURE"=2115232, "SENSOR COOLER STATUS"=2115280, "EXPOSURE TIME"=2049184, "DEFECT CORRECT MODE"=4670368, "BINNING"=4215968, "INTERNAL LINE SPEED"=4226000, "INTERNAL LINE INTERVAL"=4226016, "NUMBER OF OUTPUT TRIGGER CONNECTOR"=1852320, "OUTPUT TRIGGER SOURCE[0]"=1852576, "OUTPUT TRIGGER SOURCE[1]"=1852832, "OUTPUT TRIGGER SOURCE[2]"=1853088, "OUTPUT TRIGGER POLARITY[0]"=1852592, "OUTPUT TRIGGER POLARITY[1]"=1852848, "OUTPUT TRIGGER POLARITY[2]"=1853104, "OUTPUT TRIGGER ACTIVE[0]"=1852608, "OUTPUT TRIGGER ACTIVE[1]"=1852864, "OUTPUT TRIGGER ACTIVE[2]"=1853120, "OUTPUT TRIGGER DELAY[0]"=1852624, "OUTPUT TRIGGER DELAY[1]"=1852880, "OUTPUT TRIGGER DELAY[2]"=1853136, "OUTPUT TRIGGER PERIOD[0]"=1852640, "OUTPUT TRIGGER PERIOD[1]"=1852896, "OUTPUT TRIGGER PERIOD[2]"=1853152, "OUTPUT TRIGGER KIND[0]"=1852656, "OUTPUT TRIGGER KIND[1]"=1852912, "OUTPUT TRIGGER KIND[2]"=1853168, "OUTPUT TRIGGER BASE SENSOR[0]"=1852672, "OUTPUT TRIGGER BASE SENSOR[1]"=1852928, "OUTPUT TRIGGER BASE SENSOR[2]"=1853184, "OUTPUT TRIGGER PRE HSYNC COUNT"=1852704] ("Parameter")
            w591 = 0 items=["Snap", "Sequence"] ("Capture mode")
            w594 = u32 2049184 items=["SENSOR MODE"=4212128, "READOUT SPEED"=4211872, "READOUT DIRECTION"=4211904, "TRIGGER GLOBAL EXPOSURE"=2049680, "TRIGGER DELAY"=1066480, "INTERNAL TRIGGER HANDLING"=1066496, "SYNC READOUT SYSTEM BLANK"=1066528, "SENSOR TEMPERATURE"=2115232, "SENSOR COOLER STATUS"=2115280, "EXPOSURE TIME"=2049184, "DEFECT CORRECT MODE"=4670368, "BINNING"=4215968, "INTERNAL LINE SPEED"=4226000, "INTERNAL LINE INTERVAL"=4226016, "NUMBER OF OUTPUT TRIGGER CONNECTOR"=1852320, "OUTPUT TRIGGER SOURCE[0]"=1852576, "OUTPUT TRIGGER SOURCE[1]"=1852832, "OUTPUT TRIGGER SOURCE[2]"=1853088, "OUTPUT TRIGGER POLARITY[0]"=1852592, "OUTPUT TRIGGER POLARITY[1]"=1852848, "OUTPUT TRIGGER POLARITY[2]"=1853104, "OUTPUT TRIGGER ACTIVE[0]"=1852608, "OUTPUT TRIGGER ACTIVE[1]"=1852864, "OUTPUT TRIGGER ACTIVE[2]"=1853120, "OUTPUT TRIGGER DELAY[0]"=1852624, "OUTPUT TRIGGER DELAY[1]"=1852880, "OUTPUT TRIGGER DELAY[2]"=1853136, "OUTPUT TRIGGER PERIOD[0]"=1852640, "OUTPUT TRIGGER PERIOD[1]"=1852896, "OUTPUT TRIGGER PERIOD[2]"=1853152, "OUTPUT TRIGGER KIND[0]"=1852656, "OUTPUT TRIGGER KIND[1]"=1852912, "OUTPUT TRIGGER KIND[2]"=1853168, "OUTPUT TRIGGER BASE SENSOR[0]"=1852672, "OUTPUT TRIGGER BASE SENSOR[1]"=1852928, "OUTPUT TRIGGER BASE SENSOR[2]"=1853184, "OUTPUT TRIGGER PRE HSYNC COUNT"=1852704] ("Parameter")
            # "Timelapse"
            n337 = call <userlib>:"tm_initialize_40.vi"() -> ("error out"=w597:errorcluster)  [unwired: 8 in, 3 out]
            n338 = call <userlib>:"tm_opencamera_40.vi"("error in (no error)"=w597) -> ("error out"=w596:errorcluster, "Handle out"=w595:u32)  [unwired: 8 in, 1 out]
            n339 = local read "Binning"() -> (w581:dbl)
            n340 = call <userlib>:"tm_setarea_40.vi"("error in (no error)"=w596, "Sub Region"=w588, "Handle in"=w595) -> ("error out"=w584:errorcluster, "Handle out"=w586:u32)  [unwired: 7 in]
            n341 = call <userlib>:"tm_setparameter_40.vi"("error in (no error)"=w584, "Value in"=w581, "Parameter"=w582, "Handle in"=w586) -> ("error out"=w583:errorcluster, "Handle out"=w585:u32)  [unwired: 6 in]
            n342 = call <userlib>:"tm_setparameter_40.vi"("error in (no error)"=w583, "Value in"=w587, "Parameter"=w594, "Handle in"=w585) -> ("error out"=w593:errorcluster, "Handle out"=w592:u32)  [unwired: 6 in]
            n343 = call <userlib>:"tm_preparecapture_40.vi"("error in (no error)"=w593, "Capture mode"=w591, "Handle in"=w592) -> ("error out"=w589:errorcluster, "Handle out"=w590:u32)  [unwired: 5 in, 2 out]
            n344 = stacked-sequence {
              tunnel: w590 -> [_ w625 _]
              tunnel: w589 -> [_ w624 _]
              tunnel: w587 -> [w613 _ _]
              tunnel: w588 -> [w612 _ _]
              frame #0 {
                # "Initiaize calibration sequence"
                n345 = local read "Calibration Folder"() -> (w611:path)
                n346 = local read "LED Power"() -> (w610:dbl)
                n347 = local write "Calibrating... 2"(TRUE ("Calibrating...")) -> ()
                n348 = call <vilib>:"Check if File or Folder Exists.vi"("path"=w611) -> ("file or folder exists?"=w615:bool, "dup path"=w616:path)  [unwired: 8 in, 1 out]
                n349 = local read "Toup Crop 5440x3648"() -> (w604:T2)
                n350 = local read "ExpoGain"() -> (w602:u16)
                n351 = Cluster To Array(cluster=w612) -> (array=w605:i32[])
                n352 = case shown="False" w615 {
                  tunnel: w616 -> [w619 w620]
                  tunnel: [w618 w620] -> w614
                  frame False {
                    n353 = Create Folder(path (use dialog)=w619) -> (created path=w618:path)  [unwired: 2 in, 2 out]
                  }
                  frame True {
                  }
                }
                n354 = local read "Z depth (int)"() -> (w599:dbl)
                n355 = local read "Expotime (ms)"() -> (w598:dbl)
                n356 = local read "Z Interval (mm)"() -> (w600:dbl)
                n357 = local read "Time Interval"() -> (w606:dbl)
                n358 = local read "TimeY"() -> (w608:dbl)
                n359 = local read "TimeX"() -> (w609:dbl)
                n360 = local read "TimeZ"() -> (w607:dbl)
                n361 = local read "Binning"() -> (w601:dbl)
                n362 = Cluster To Array(cluster=w604) -> (array=w603:i32[])
                n363 = script code="saveTimeMetafile;"("path"=w614, "orcaExp"=w613, "LEDPower"=w610, "TimeInterval"=w606, "TimeZ"=w607, "TimeY"=w608, "TimeX"=w609, "AmExp"=w598, "OrcaCrop"=w605, "AmCrop"=w603, "AmGain"=w602, "binning"=w601, "Zdepth"=w599, "Zinterval"=w600) -> ()  [unwired: 1 in, 1 out]
              }
              frame #1 {
                # "Calibration sequence"
                n364 = Subtract(x="TimeFrames", y=1.0) -> (x-y=w622:dbl)
                n365 = for {
                  N: w622 -> [_]
                  tunnel: w625 -> [w628]
                  tunnel: w624 -> [w627]
                  i -> [w626]
                  stop <- w629 stop-if-true
                  n366 = flat-sequence {
                    tunnel: [w634] -> w629
                    tunnel: w628 -> [w633]
                    tunnel: w627 -> [w632]
                    tunnel: w626 -> [w631]
                    frame #0 {
                      n367 = for {
                        N: "Z depth (int)" -> [_]
                        tunnel: [w641] -> w634
                        tunnel: w633 -> [w640]
                        tunnel: w632 -> [w639]
                        tunnel: w631 -> [w638]
                        i -> [w635]
                        n368 = Add(x=1, y=w638) -> (x+y=w636:i32)
                        "Count 2" <- w636
                        n369 = stacked-sequence {
                          tunnel: [_ _ _ _ _ _ "Abort 3"] -> w641
                          tunnel: w639 -> [_ _ _ _ w678 w695 _]
                          tunnel: w640 -> [_ _ _ _ w679 w696 w719]
                          tunnel: w636 -> [_ _ _ _ _ w694 _]
                          tunnel: w635 -> [_ _ w662 _ _ w692 _]
                          frame #0 {
                            # "Change x axis location of point source"
                            n370 = global read "callback_Done.vi" "X Motor Reference"() -> (w645:refnum<k7>)
                            n371 = invoke class="MG17Motor" method="MoveAbsoluteEnc"(reference=w645, "lChanID"=0, "fAbsPosCh1"="TimeX", "fAbsPosCh2"="TimeX", "lTimeInc"=1000, "bWait"=FALSE) -> ("fAbsPosCh1"=→"X Pos (mm) 3":sgl)  [unwired: 2 in, 7 out]
                            n372 = global write "callback_Done.vi" "X Motor done"(FALSE ("Motor done")) -> ()
                            n373 = Wait (ms)(milliseconds to wait=0) -> ()  [unwired: 1 out]
                            "Moving... 3" <- TRUE ("Waiting...")
                          }
                          frame #1 {
                            # "Change y axis location of point source"
                            n374 = global read "callback_Done.vi" "Y Motor Reference"() -> (w654:refnum<k7>)
                            n375 = Wait (ms)(milliseconds to wait=0) -> ()  [unwired: 1 out]
                            n376 = invoke class="MG17Motor" method="MoveAbsoluteEnc"(reference=w654, "lChanID"=0, "fAbsPosCh1"="TimeY", "fAbsPosCh2"="TimeY", "lTimeInc"=1000, "bWait"=FALSE) -> ("fAbsPosCh1"=→"Y Pos (mm) 3":sgl)  [unwired: 2 in, 7 out]
                            n377 = global write "callback_Done.vi" "Y Motor done"(FALSE ("Motor done")) -> ()
                          }
                          frame #2 {
                            # "Change z axis location of point source, if needed"
                            n378 = Multiply(x=w662, y="Z Interval (mm)") -> (x*y=w661:dbl)
                            n379 = local read "Shrink"() -> (w664:dbl)
                            n380 = Add(x="TimeZ", y=w661) -> (x+y=w659:dbl)
                            n381 = Add(x=w664, y=w659) -> (x+y=w665:dbl)
                            n382 = global read "callback_Done.vi" "Z Motor Reference"() -> (w668:refnum<k7>)
                            n383 = invoke class="MG17Motor" method="MoveAbsoluteEnc"(reference=w668, "lChanID"=0, "fAbsPosCh1"=w665, "fAbsPosCh2"=w665, "lTimeInc"=1000, "bWait"=FALSE) -> ("fAbsPosCh1"=→"Z Pos (mm) 3":sgl)  [unwired: 2 in, 7 out]
                            n384 = global write "callback_Done.vi" "Z Motor done"(FALSE ("Motor done")) -> ()
                          }
                          frame #3 {
                            # "(If moving) Wait until X,Y,Z motion is finished."
                            n385 = while {
                              stop <- w673 stop-if-true
                              n386 = global read "callback_Done.vi" "Z Motor done"() -> (w677:bool)
                              n387 = global read "callback_Done.vi" "Y Motor done"() -> (w675:bool)
                              n388 = global read "callback_Done.vi" "X Motor done"() -> (w674:bool)
                              n389 = And(x=w675, y=w674) -> (x .and. y?=w676:bool)
                              n390 = And(x=w677, y=w676) -> (x .and. y?=w673:bool)
                            }
                            n391 = Wait (ms)(milliseconds to wait=100) -> ()  [unwired: 1 out]
                          }
                          frame #4 {
                            # "Throw one frame out"
                            n392 = flat-sequence {
                              tunnel: w679 -> [w686]
                              tunnel: w678 -> [w681]
                              frame #0 {
                                n393 = call <userlib>:"tm_startcapture_40.vi"("error in (no error)"=w681, "Handle in"=w686) -> ("error out"=w682:errorcluster, "Handle out"=w685:u32)  [unwired: 8 in]
                                n394 = call <userlib>:"tm_waitnextframe_40.vi"("error in (no error)"=w682, "Handle in"=w685) -> ("error out"=w688:errorcluster, "Frame Index"=w687:i32, "Handle out"=w689:u32)  [unwired: 6 in, 1 out]
                                n395 = call <userlib>:"tm_getframe16_40.vi"("error in (no error)"=w688, "Frame Index"=w687, "Handle in"=w689) -> ("error out"=w683:errorcluster, "Handle out"=w684:u32)  [unwired: 5 in, 2 out]
                                n396 = call <userlib>:"tm_stopcapture_40.vi"("error in (no error)"=w683, "Handle in"=w684) -> ("error out"=w680:errorcluster)  [unwired: 8 in, 1 out]
                                n397 = local write "Error Surf 2"(w680) -> ()
                              }
                              frame #1 {
                              }
                              frame #2 {
                                n398 = call <userlib>:"U3 eDAC Example.vi"("Voltage"=5.0) -> ()  [unwired: 10 in, 1 out]
                              }
                              frame #3 {
                                n399 = Wait (ms)(milliseconds to wait=u32 1000) -> ()  [unwired: 1 out]
                              }
                            }
                          }
                          frame #5 {
                            # "Capture and save HDR image"
                            n400 = for {
                              N: "FrameAve2" -> [_]
                              tunnel: w696 -> [w711]
                              tunnel: w695 -> [w704]
                              tunnel: w694 -> [w699]
                              tunnel: w692 -> [w697]
                              i -> [w698]
                              w712 = T6 1 items=["no dialog", "OK message", "continue or stop message", "OK message + warnings", "continue/stop + warnings"] ("type of dialog (OK msg:1)")
                              n401 = call <userlib>:"tm_startcapture_40.vi"("error in (no error)"=w704, "Handle in"=w711) -> ("error out"=w705:errorcluster, "Handle out"=w710:u32)  [unwired: 8 in]
                              n402 = property on="objRef" class="IntGraph (strict)"() -> ("Value"=w700:u8[][])  [unwired: 2 in, 2 out]
                              n403 = call <userlib>:"tm_waitnextframe_40.vi"("error in (no error)"=w705, "Handle in"=w710) -> ("error out"=w706:errorcluster, "Frame Index"=w703:i32, "Handle out"=w709:u32)  [unwired: 6 in, 1 out]
                              n404 = local write "Moving... 3"(FALSE ("Waiting...")) -> ()
                              n405 = Format Into String(format string="%d", w699) -> (resulting string=w714:string)  [unwired: 2 in, 1 out]
                              n406 = call <userlib>:"tm_getframe16_40.vi"("error in (no error)"=w706, "Frame Index"=w703, "Handle in"=w709) -> ("error out"=w707:errorcluster, "Data"=w702:u16[][], "Handle out"=w708:u32)  [unwired: 5 in, 1 out]
                              n407 = local write "Image"(w702) -> ()
                              n408 = call <userlib>:"tm_stopcapture_40.vi"("error in (no error)"=w707, "Handle in"=w708) -> ("error out"=w701:errorcluster)  [unwired: 8 in, 1 out]
                              n409 = script code="Frame = num2str(Frame);\nZstack = num2str(Zstack);\nUnderscore = '_';\nname = [CapPos Underscore Frame Underscore Zstack];\nsave([path,'/',name],'objCCM','objRef','xPos','yPos','zPos');"("CapPos"=w714, "objRef"=w700, "objCCM"=w702, "Frame"=w698, "Zstack"=w697) -> ("??"=w713:errorcluster)  [unwired: 1 in]
                              n410 = local write "Error Surf 2"(w701) -> ()
                              n411 = call <vilib>:"Simple Error Handler.vi"("type of dialog (OK msg:1)"=w712, "error in (no error)"=w713) -> ()  [unwired: 3 in, 5 out]
                              "Capturing" <- TRUE ("Acquiring...")
                            }
                          }
                          frame #6 {
                            # "Calculate calibration frame rate and display."
                            n412 = local write "Capturing"(FALSE ("Saving...")) -> ()
                            n413 = case shown="True" "Abort 3" {
                              tunnel: w719 -> [_ w724]
                              frame False {
                              }
                              frame True {
                                n414 = call <userlib>:"tm_unpreparecapture_40.vi"("Handle in"=w724) -> ("error out"=w723:errorcluster, "Handle out"=w722:u32)  [unwired: 9 in]
                                n415 = call <userlib>:"tm_closecamera_40.vi"("error in (no error)"=w723, "Handle in"=w722) -> ("error out"=w721:errorcluster)  [unwired: 9 in]
                                n416 = call <userlib>:"tm_deinitialize_40.vi"("error in (no error)"=w721) -> ()  [unwired: 10 in, 1 out]
                              }
                            }
                          }
                        }
                      }
                    }
                    frame #1 {
                      n417 = call <userlib>:"U3 eDAC Example.vi"("Voltage"=0.0) -> ()  [unwired: 10 in, 1 out]
                      n418 = Wait (ms)(milliseconds to wait="Time Interval") -> ()  [unwired: 1 out]
                    }
                  }
                }
              }
              frame #2 {
                w729 = u16 6 items=["Wait", "Acquire Live", "Acquire Single", "Terminate", "Calibration", "Macro", "Wait Prep"] ("Imaging status")
                # "Wrap up the calibration"
                n419 = local write "Calibrating... 2"(FALSE ("Calibrating...")) -> ()
                n420 = local write "Abort 3"(FALSE ("Abort")) -> ()
                n421 = local write "Generate Surface & Go"(FALSE) -> ()
                n422 = local write "Imaging status"(w729) -> ()
                n423 = call <userlib>:"U3 eDAC Example.vi"("Voltage"=0.0) -> ()  [unwired: 10 in, 1 out]
              }
            }
          }
          frame 6 {
            w741 = 0 items=["Snap", "Sequence"] ("Capture mode")
            w751 = u16 0 items=["Wait", "Acquire Live", "Acquire Single", "Terminate"] ("Imaging status")
            n424 = call <userlib>:"tm_initialize_40.vi"() -> ("error out"=w743:errorcluster)  [unwired: 8 in, 3 out]
            n425 = local write "Imaging status"(w751) -> ()
            n426 = call <userlib>:"tm_opencamera_40.vi"("error in (no error)"=w743) -> ("error out"=w744:errorcluster, "Handle out"=w742:u32)  [unwired: 8 in, 1 out]
            n427 = call <userlib>:"tm_preparecapture_40.vi"("error in (no error)"=w744, "Capture mode"=w741, "Handle in"=w742) -> ("error out"=w745:errorcluster, "Handle out"=w746:u32)  [unwired: 5 in, 2 out]
            n428 = call <userlib>:"tm_startcapture_40.vi"("error in (no error)"=w745, "Handle in"=w746) -> ("error out"=w748:errorcluster, "Handle out"=w747:u32)  [unwired: 8 in]
            n429 = call <userlib>:"tm_waitnextframe_40.vi"("error in (no error)"=w748, "Handle in"=w747) -> ("error out"=w740:errorcluster, "Frame Index"=w739:i32, "Handle out"=w738:u32)  [unwired: 6 in, 1 out]
            n430 = call <userlib>:"tm_getframe16_40.vi"("error in (no error)"=w740, "Frame Index"=w739, "Handle in"=w738) -> ("error out"=w736:errorcluster, "Handle out"=w737:u32)  [unwired: 5 in, 2 out]
            n431 = call <userlib>:"tm_stopcapture_40.vi"("error in (no error)"=w736, "Handle in"=w737) -> ("error out"=w750:errorcluster, "Handle out"=w749:u32)  [unwired: 8 in]
            n432 = call <userlib>:"tm_unpreparecapture_40.vi"("error in (no error)"=w750, "Handle in"=w749) -> ("error out"=w734:errorcluster, "Handle out"=w735:u32)  [unwired: 8 in]
            n433 = call <userlib>:"tm_closecamera_40.vi"("error in (no error)"=w734, "Handle in"=w735) -> ("error out"=w733:errorcluster)  [unwired: 9 in]
            n434 = call <userlib>:"tm_deinitialize_40.vi"("error in (no error)"=w733) -> ("error out"=→"Error Out Wait":errorcluster)  [unwired: 10 in]
          }
        }
      }
      n435 = while {
        tunnel: w73 -> [w753]
        tunnel: w72 -> [w752]
        stop <- w756 stop-if-true
        w755 = T6 1 items=["no dialog", "OK message", "continue or stop message", "OK message + warnings", "continue/stop + warnings"] ("type of dialog (OK msg:1)")
        n436 = event shown="[7] \"Save image for pix2pix\": Value Change" {
          selector: w753 -> [_ _ _ _ _ _ _ _ _ _ _ _ _ _ _ _ _ _ _ _ _ _ _ _ _ _ _ _ _ _ _ _ _ _ _ _ _ _ _ _ _]
          dyn-events: _ -> [_ _ _ _ _ _ _ _ _ _ _ _ _ _ _ _ _ _ _ _ _ _ _ _ _ _ _ _ _ _ _ _ _ _ _ _ _ _ _ _ _]
          timeout: 10 -> [_ _ _ _ _ _ _ _ _ _ _ _ _ _ _ _ _ _ _ _ _ _ _ _ _ _ _ _ _ _ _ _ _ _ _ _ _ _ _ _ _]
          tunnel: [_ TRUE ("Stop") _ _ _ _ _ _ _ _ _ _ _ _ _ _ _ _ _ _ _ _ _ _ _ _ _ _ _ _ _ _ _ _ _ _ _ _ _ _ _] -> w756
          tunnel: [_ _ w774 w776 _ _ _ _ _ _ _ _ _ _ _ _ _ _ w882 _ w889 w892 w905 _ _ _ _ _ _ _ _ _ _ _ _ _ _ _ _ _ _] -> w754
          tunnel: w752 -> [_ _ _ _ _ _ _ _ _ _ _ _ _ _ _ _ _ _ _ _ _ _ _ _ _ _ _ _ _ _ _ _ _ _ _ w933 w973 w974 w976 _ _]
          event Timeout {
            n437 = event-data() -> ()  [unwired: 1 in, 2 out]
            n438 = global read "callback_Done.vi" "X Motor Reference"() -> (w765:refnum<k7>)
            n439 = global read "callback_Done.vi" "Y Motor Reference"() -> (w768:refnum<k7>)
            n440 = global read "callback_Done.vi" "Z Motor Reference"() -> (w762:refnum<k7>)
            n441 = invoke class="MG17Motor" method="GetPosition"(reference=w765, "lChanID"=0, "pfPosition"=sgl 0.0) -> ("pfPosition"=w759:sgl)  [unwired: 2 in, 4 out]
            "xPos" <- w759
            n442 = invoke class="MG17Motor" method="GetPosition"(reference=w768, "lChanID"=0, "pfPosition"=sgl 0.0) -> ("pfPosition"=w758:sgl)  [unwired: 2 in, 4 out]
            "yPos" <- w758
            n443 = invoke class="MG17Motor" method="GetPosition"(reference=w762, "lChanID"=0, "pfPosition"=sgl 0.0) -> ("pfPosition"=w760:sgl)  [unwired: 2 in, 4 out]
            "zPos" <- w760
            n444 = script code="MATLAB script"("xPos"=w759, "yPos"=w758, "zPos"=w760) -> ()  [unwired: 1 in, 1 out]
          }
          event "Stop": Value Change {
            w772 = u16 3 items=["Wait", "Acquire Single", "Acquire Live", "Terminate"] ("Imaging status")
            # "Properly terminate all hardware controls here\n ex> All kidns of camera, Thorlab stage, etc."
            n445 = event-data() -> ()  [unwired: 1 in, 5 out]
            n446 = local write "Imaging status"(w772) -> ()
            n447 = local write "Grab"(FALSE ("Grab")) -> ()
            n448 = call <userlib>:"U3 eDAC Example.vi"("Voltage"=0.0) -> ()  [unwired: 10 in, 1 out]
          }
          event "Load Cal": Mouse Up {
            n449 = event-data() -> ()  [unwired: 1 in, 7 out]
            n450 = call "File Dialog"() -> ("selected path"=w775:path)  [unwired: 12 in, 3 out]
            n451 = script code="if exist(filename, 'file') == 2\n   calPath = filename;\n   load(calPath);\n   calibration.A           = A;\n   calibration.U           = U;\n   calibration.s            = s;\n   calibration.V           = V;\n   calibration.DC         = DC;\n   calibration.calID            = calID;\n   calibration.imgFOV      = imgFOV;\n   calibration.objFOV        = objFOV;\n   calibration.objFOVInd  = find(objFOV==1);\n   calibration.zSize            = zSize;\n   calibration.psfSize         = psfSize;\n   calibration.normArray  = normArray;  \nend\n\nclear A U s V DC calID imgFOV objFOV ... \n          objFOVInd zSize psfSize normArray"("filename"=w775) -> ("??"=w774:errorcluster)  [unwired: 1 in]
          }
          event "Save Data": Mouse Up {
            n452 = event-data() -> ()  [unwired: 1 in, 7 out]
            n453 = call "Save Dialog"("start path"="Workspace") -> ("selected path"=w777:path)  [unwired: 11 in, 3 out]
            n454 = script code="if ~strcmp(filename,'<Not A Path>')\n   saveData;\nend"("filename"=w777) -> ("??"=w776:errorcluster)  [unwired: 1 in]
          }
          event "Play": Mouse Up {
            n455 = event-data() -> ()  [unwired: 1 in, 7 out]
            n456 = local read "Imaging status"() -> (w779:u16)
            n457 = case shown="0" w779 {
              frame 0 {
                n458 = stacked-sequence {
                  frame #0 {
                    w785 = 1 items=["Snap", "Sequence"] ("Capture mode")
                    n459 = global read "GlobalVariables.vi" "Orca Handle"() -> (w780:u32)
                    n460 = call <userlib>:"tm_preparecapture.vi"("Frames"=1, "Capture mode"=w785, "Handle in"=w780) -> ("error out"=w783:errorcluster, "Buffer Info"=w781:T8, "Handle out"=w782:u32)  [unwired: 5 in, 1 out]
                    n461 = call <userlib>:"tm_startcapture_b.vi"("error in (no error)"=w783, "Handle in"=w782) -> ()  [unwired: 8 in, 2 out]
                    n462 = global write "GlobalVariables.vi" "Orca Buffer"(w781) -> ()
                  }
                  frame #1 {
                    w786 = u16 1 items=["Wait", "Acquire Live", "Acquire Single", "Terminate"] ("Imaging status")
                    n463 = local write "Imaging status"(w786) -> ()
                  }
                }
              }
              frame 1, Default {
                n464 = call "Display Message to User2"() -> ()  [unwired: 10 in, 2 out]
              }
            }
          }
          event "Pause": Mouse Up {
            n465 = event-data() -> ()  [unwired: 1 in, 7 out]
            n466 = local read "Imaging status"() -> (w787:u16)
            n467 = case shown="1" w787 {
              frame 0, Default {
              }
              frame 1 {
                w788 = u16 6 items=["Wait", "Acquire Live", "Acquire Single", "Terminate", "Calibration", "Macro", "Wait Prep"] ("Imaging status")
                n468 = local write "Imaging status"(w788) -> ()
              }
            }
          }
          event "Single": Mouse Up {
            n469 = event-data() -> ()  [unwired: 1 in, 7 out]
            n470 = local read "Imaging status"() -> (w790:u16)
            n471 = Less Or Equal?(x=w790, y=u16 2) -> (x <= y?=w791:bool)
            n472 = case shown="False" w791 {
              frame False {
                n473 = call "Display Message to User3"() -> ()  [unwired: 10 in, 2 out]
              }
              frame True {
                n474 = stacked-sequence {
                  frame #0 {
                    w792 = 1 items=["Snap", "Sequence"] ("Capture mode")
                    n475 = global read "GlobalVariables.vi" "Orca Handle"() -> (w797:u32)
                    n476 = call <userlib>:"tm_preparecapture.vi"("Frames"=1, "Capture mode"=w792, "Handle in"=w797) -> ("error out"=w794:errorcluster, "Buffer Info"=w796:T8, "Handle out"=w795:u32)  [unwired: 5 in, 1 out]
                    n477 = call <userlib>:"tm_startcapture_b.vi"("error in (no error)"=w794, "Handle in"=w795) -> ()  [unwired: 8 in, 2 out]
                    n478 = global write "GlobalVariables.vi" "Orca Buffer"(w796) -> ()
                  }
                  frame #1 {
                    w798 = u16 2 items=["Wait", "Acquire Live", "Acquire Single", "Terminate"] ("Imaging status")
                    n479 = local write "Imaging status"(w798) -> ()
                  }
                }
              }
            }
          }
          event "Save image for pix2pix": Value Change {
            n480 = event-data() -> ()  [unwired: 1 in, 6 out]
            n481 = local read "Image"() -> (w801:u16[][])
            n482 = local read "objRef"() -> (w800:u8[][])
            n483 = script code="save('C:\\Cannula Microscope\\realtime\\realtime.mat', 'objCCM', 'objRef');\npythonScriptPath = 'C:\\Users\\menon\\pytorch-CycleGAN-and-pix2pix\\realtime_test.py';\ncommandStr = ['python \"', pythonScriptPath, '\"'];\nsystem(commandStr);\n\n%FakePix2pix =[];\n%FakePix2Pix = realtimePix2Pix();\n%FakePix2pix = FakePix2pix(:);\n%image(FakePix2Pix)\n%colormap gray" ("Script Node")("objRef"=w800, "objCCM"=w801) -> ("??"=w799:errorcluster)  [unwired: 1 in, 1 out]
            n484 = local write "Error Out Wait"(w799) -> ()
            n485 = disable-structure shown="Disabled" {
              disable-tunnel: _ -> [w805 _]
              frame Disabled {
                n486 = Reshape Array(w805, 256 ("dimension size"), 256 ("dimension size")) -> (w802:void[][])
                n487 = Array To Cluster() -> ()  [unwired: 1 in, 1 out]
                n488 = local write "Image 2"(w802) -> ()
              }
              frame Enabled {
              }
            }
          }
          event "Start Realtime\npix2pix": Value Change {
            n489 = event-data() -> ()  [unwired: 1 in, 6 out]
            n490 = script code="stopFlagPath = 'C:\\Cannula Microscope\\realtime\\stopFlag.txt';\nif isfile(stopFlagPath)\n    delete(stopFlagPath);\n    disp('Stop flag deleted.');\nelse\n    disp('Stop flag does not exist.');\nend\n\nFakePix2Pix = realtimePix2Pix();" ("Script Node")() -> ()  [unwired: 1 in, 1 out]
          }
          event "Stop Realtime\npix2pix": Value Change {
            n491 = event-data() -> ()  [unwired: 1 in, 6 out]
            n492 = script code="stopFlagPath = 'C:\\Cannula Microscope\\realtime\\stopFlag.txt';\nfileID = fopen(stopFlagPath, 'w');\nfclose(fileID);\ndisp('Stop flag created.');" ("Script Node")() -> ()  [unwired: 1 in, 1 out]
          }
          event "Start Cal": Mouse Up {
            n493 = event-data() -> ()  [unwired: 1 in, 7 out]
            n494 = local read "Imaging status"() -> (w806:u16)
            n495 = case shown="0" w806 {
              frame 0 {
                w807 = u16 4 items=["Wait", "Acquire Live", "Acquire Single", "Terminate", "Calibration"] ("Imaging status")
                n496 = local write "Imaging status"(w807) -> ()
              }
              frame 1, Default {
                n497 = call "Display Message to User4"() -> ()  [unwired: 10 in, 2 out]
              }
            }
          }
          event "Kinetic Series": Value Change {
            n498 = event-data() -> ()  [unwired: 1 in, 5 out]
            n499 = case shown="True" "Kinetic Series" {
              frame False {
                n500 = script code="f = 0;\nsaveMode = 'single';"() -> ()  [unwired: 1 in, 1 out]
              }
              frame True {
                n501 = script code="f = 0;\nsaveMode = 'series';"() -> ()  [unwired: 1 in, 1 out]
              }
            }
          }
          event "Save Support": Value Change {
            n502 = event-data() -> ()  [unwired: 1 in, 6 out]
            n503 = flat-sequence {
              frame #0 {
                n504 = global read "callback_Done.vi" "X Motor Reference"() -> (w822:refnum<k7>)
                n505 = global read "callback_Done.vi" "Y Motor Reference"() -> (w825:refnum<k7>)
                n506 = global read "callback_Done.vi" "Z Motor Reference"() -> (w819:refnum<k7>)
                n507 = invoke class="MG17Motor" method="GetPosition"(reference=w822, "lChanID"=0, "pfPosition"=sgl 0.0) -> ("pfPosition"=w812:sgl)  [unwired: 2 in, 4 out]
                "xPos 2" <- w812
                n508 = invoke class="MG17Motor" method="GetPosition"(reference=w825, "lChanID"=0, "pfPosition"=sgl 0.0) -> ("pfPosition"=w813:sgl)  [unwired: 2 in, 4 out]
                "yPos 2" <- w813
                n509 = invoke class="MG17Motor" method="GetPosition"(reference=w819, "lChanID"=0, "pfPosition"=sgl 0.0) -> ("pfPosition"=w814:sgl)  [unwired: 2 in, 4 out]
                "zPos 2" <- w814
                n510 = script code="[m,n] = size(Support);\nN = n +1;\nSupport(:,N) = [xSup ySup zSup];\nXSup(N) = xSup;\nYSup(N) = ySup;"("xSup"=w812, "ySup"=w813, "zSup"=w814) -> ("XSup"=w811:dbl[], "YSup"=w810:dbl[], "N"=→"PointNumber":dbl)  [unwired: 1 in, 1 out]
                n511 = call "Convert to Dynamic Data"("Array"=w811) -> ("Dynamic Data Type"=w816:dynamicdata)  [unwired: 3 in]
                n512 = call "Convert to Dynamic Data2"("Array"=w810) -> ("Dynamic Data Type"=w815:dynamicdata)  [unwired: 3 in]
                n513 = call "Build XY Graph"("Y Input"=w815, "X Input"=w816) -> ("XY Graph"=→"XY Graph":cluster{"X":dbl[], "Y":dbl[]}[])  [unwired: 8 in, 1 out]
              }
              frame #1 {
                n514 = local write "Save Support"(FALSE) -> ()
              }
            }
          }
          event "Update Support Graph": Value Change {
            n515 = event-data() -> ()  [unwired: 1 in, 6 out]
            n516 = flat-sequence {
              frame #0 {
                n517 = script code="for i = 1:length(Support)\nXSup(i) = Support(1,i);\nYSup(i) = Support(2,i);\nend"() -> ("XSup"=w832:dbl[], "YSup"=w829:dbl[])  [unwired: 1 in, 1 out]
                n518 = call "Convert to Dynamic Data5"("Array"=w832) -> ("Dynamic Data Type"=w831:dynamicdata)  [unwired: 3 in]
                n519 = call "Convert to Dynamic Data6"("Array"=w829) -> ("Dynamic Data Type"=w830:dynamicdata)  [unwired: 3 in]
                n520 = call "Build XY Graph3"("Y Input"=w830, "X Input"=w831) -> ("XY Graph"=w828:cluster{"X":dbl[], "Y":dbl[]}[])  [unwired: 8 in, 1 out]
                n521 = local write "XY Graph"(w828) -> ()
              }
              frame #1 {
                n522 = local write "Update Support Graph"(FALSE) -> ()
              }
            }
          }
          event "Clear Support": Value Change {
            n523 = event-data() -> ()  [unwired: 1 in, 6 out]
            n524 = flat-sequence {
              frame #0 {
                n525 = script code="N = [];\nSupport = [];\nXSup = [];\nYSup = [];\nxSup = [];\nySup = [];\nzSup = [];\nxRep = [];\nyRep = [];\nzRep = [];"() -> ("XSup"=w837:dbl[], "YSup"=w836:dbl[])  [unwired: 1 in, 1 out]
                n526 = call "Convert to Dynamic Data4"("Array"=w836) -> ("Dynamic Data Type"=w839:dynamicdata)  [unwired: 3 in]
                n527 = call "Convert to Dynamic Data3"("Array"=w837) -> ("Dynamic Data Type"=w838:dynamicdata)  [unwired: 3 in]
                n528 = call "Build XY Graph2"("Y Input"=w839, "X Input"=w838) -> ("XY Graph"=w835:cluster{"X":dbl[], "Y":dbl[]}[])  [unwired: 8 in, 1 out]
                n529 = local write "PointNumber"(0.0 ("PointNumber")) -> ()
                n530 = local write "XY Graph"(w835) -> ()
              }
              frame #1 {
                n531 = local write "Clear Support"(FALSE) -> ()
              }
            }
          }
          event "Generate Surface & Go": Value Change {
            n532 = event-data() -> ()  [unwired: 1 in, 6 out]
            n533 = flat-sequence {
              frame #0 {
                n534 = call <userlib>:"tm_initialize_40.vi"() -> ("error out"=w858:errorcluster)  [unwired: 8 in, 3 out]
                n535 = call <userlib>:"tm_opencamera_40.vi"("error in (no error)"=w858) -> ("error out"=w857:errorcluster, "Handle out"=w856:u32)  [unwired: 8 in, 1 out]
                n536 = call <userlib>:"tm_preparecapture_40.vi"("error in (no error)"=w857, "Handle in"=w856) -> ("error out"=w855:errorcluster, "Handle out"=w854:u32)  [unwired: 6 in, 2 out]
                n537 = call <userlib>:"tm_startcapture_40.vi"("error in (no error)"=w855, "Handle in"=w854) -> ("error out"=w853:errorcluster, "Handle out"=w852:u32)  [unwired: 8 in]
                n538 = call <userlib>:"tm_waitnextframe_40.vi"("error in (no error)"=w853, "Handle in"=w852) -> ("error out"=w851:errorcluster, "Frame Index"=w850:i32, "Handle out"=w849:u32)  [unwired: 6 in, 1 out]
                n539 = call <userlib>:"tm_getframe16_40.vi"("error in (no error)"=w851, "Frame Index"=w850, "Handle in"=w849) -> ("error out"=w848:errorcluster, "Handle out"=w847:u32)  [unwired: 5 in, 2 out]
                n540 = call <userlib>:"tm_stopcapture_40.vi"("error in (no error)"=w848, "Handle in"=w847) -> ("error out"=w846:errorcluster, "Handle out"=w845:u32)  [unwired: 8 in]
                n541 = call <userlib>:"tm_unpreparecapture_40.vi"("error in (no error)"=w846, "Handle in"=w845) -> ("error out"=w844:errorcluster, "Handle out"=w843:u32)  [unwired: 8 in]
                n542 = call <userlib>:"tm_closecamera_40.vi"("error in (no error)"=w844, "Handle in"=w843) -> ("error out"=w842:errorcluster)  [unwired: 9 in]
                n543 = call <userlib>:"tm_deinitialize_40.vi"("error in (no error)"=w842) -> ("error out"=→"Error Out Surf Prep":errorcluster)  [unwired: 10 in]
              }
              frame #1 {
                n544 = local read "Imaging status"() -> (w859:u16)
                n545 = case shown="0" w859 {
                  frame 0 {
                    n546 = local write "Imaging status"(u16 5 ("Imaging status")) -> ()
                  }
                  frame 1, Default {
                    n547 = call "Display Message to User"() -> ()  [unwired: 10 in, 2 out]
                  }
                }
              }
            }
          }
          event "StartShrinking": Value Change {
            n548 = event-data() -> ()  [unwired: 1 in, 6 out]
          }
          event "Start Timelapse": Value Change {
            n549 = event-data() -> ()  [unwired: 1 in, 6 out]
            n550 = flat-sequence {
              frame #0 {
                n551 = call <userlib>:"tm_initialize_40.vi"() -> ("error out"=w878:errorcluster)  [unwired: 8 in, 3 out]
                n552 = call <userlib>:"tm_opencamera_40.vi"("error in (no error)"=w878) -> ("error out"=w877:errorcluster, "Handle out"=w876:u32)  [unwired: 8 in, 1 out]
                n553 = call <userlib>:"tm_preparecapture_40.vi"("error in (no error)"=w877, "Handle in"=w876) -> ("error out"=w875:errorcluster, "Handle out"=w874:u32)  [unwired: 6 in, 2 out]
                n554 = call <userlib>:"tm_startcapture_40.vi"("error in (no error)"=w875, "Handle in"=w874) -> ("error out"=w873:errorcluster, "Handle out"=w872:u32)  [unwired: 8 in]
                n555 = call <userlib>:"tm_waitnextframe_40.vi"("error in (no error)"=w873, "Handle in"=w872) -> ("error out"=w871:errorcluster, "Frame Index"=w870:i32, "Handle out"=w869:u32)  [unwired: 6 in, 1 out]
                n556 = call <userlib>:"tm_getframe16_40.vi"("error in (no error)"=w871, "Frame Index"=w870, "Handle in"=w869) -> ("error out"=w868:errorcluster, "Handle out"=w867:u32)  [unwired: 5 in, 2 out]
                n557 = call <userlib>:"tm_stopcapture_40.vi"("error in (no error)"=w868, "Handle in"=w867) -> ("error out"=w866:errorcluster, "Handle out"=w865:u32)  [unwired: 8 in]
                n558 = call <userlib>:"tm_unpreparecapture_40.vi"("error in (no error)"=w866, "Handle in"=w865) -> ("error out"=w864:errorcluster, "Handle out"=w863:u32)  [unwired: 8 in]
                n559 = call <userlib>:"tm_closecamera_40.vi"("error in (no error)"=w864, "Handle in"=w863) -> ("error out"=w862:errorcluster)  [unwired: 9 in]
                n560 = call <userlib>:"tm_deinitialize_40.vi"("error in (no error)"=w862) -> ("error out"=→"Error Out Surf Prep 2":errorcluster)  [unwired: 10 in]
              }
              frame #1 {
                n561 = local read "Imaging status"() -> (w879:u16)
                n562 = case shown="0" w879 {
                  frame 0 {
                    n563 = local write "Imaging status"(u16 7 ("Imaging status")) -> ()
                  }
                  frame 1, Default {
                    n564 = call "Display Message to User5"() -> ()  [unwired: 10 in, 2 out]
                  }
                }
              }
            }
          }
          event "Frame Ave Count": Value Change {
            n565 = event-data() -> ("NewVal"=w883:dbl)  [unwired: 1 in, 4 out]
            n566 = script code="imgRaw = frames(f).imgRaw;\n   imgPro  = frames(f).imgPro;\n   objProZ = frames(f).objPro(:,:,zInd);"("f"=w883) -> ("??"=w882:errorcluster, "imgPro"=w881:dbl[][])  [unwired: 1 in, 1 out]
            n567 = local write "imgPro"(w881) -> ()
          }
          event "Z Index": Value Change {
            w886 = T6 1 items=["no dialog", "OK message", "continue or stop message", "OK message + warnings", "continue/stop + warnings"] ("type of dialog (OK msg:1)")
            n568 = event-data() -> ()  [unwired: 1 in, 5 out]
            n569 = script code="if zInd < 1\n      zInd = 1;\n   elseif zInd > zSize\n      zInd = zSize;\n   end"("zInd"="Z Index") -> ("??"=w885:errorcluster, "f"=w884:dbl)  [unwired: 1 in]
            n570 = property on="Frame Ave Count" class="DigNum (strict)"("Val(Sgnl)"=w884) -> ()  [unwired: 2 in, 2 out]
            n571 = call <vilib>:"Simple Error Handler.vi"("type of dialog (OK msg:1)"=w886, "error in (no error)"=w885) -> ()  [unwired: 3 in, 5 out]
          }
          event "Shift input X", "Shift Y": Value Change {
            n572 = event-data() -> ()  [unwired: 1 in, 5 out]
            n573 = script code="frames(f).sfX = sfX;\n    frames(f).sfY = sfY;\n    \n    processImage;\n    reconstructObject;\n    processObject;\n    \n    imgPro = frames(f).imgPro;\n    objProZ = frames(f).objPro(:,:,zInd);"("sfX"="Shift input X", "sfY"="Shift Y") -> ("??"=w889:errorcluster, "imgPro"=w888:dbl[][])  [unwired: 1 in, 1 out]
            n574 = local write "imgPro"(w888) -> ()
          }
          event "Ctrl Factor", "Method": Value Change {
            n575 = event-data() -> ()  [unwired: 1 in, 5 out]
            n576 = script code="frames(f).method = method;\n frames(f).ctrlFactor = ctrlFactor;\n\n    reconstructObject;   \n    processObject;\n    \n objProZ = frames(f).objPro(:,:,zInd);"("ctrlFactor"="Ctrl Factor", "method"="Method") -> ("??"=w892:errorcluster)  [unwired: 1 in, 1 out]
          }
          event "Gain", "Brigtness", "Threshold", "Convolution", "Mask size (%)", "Mask Shift X", "Mask Shift Y", "Masking": Value Change {
            n577 = event-data() -> ()  [unwired: 1 in, 5 out]
            n578 = Boolean To (0,1)(Boolean="Masking") -> (0, 1=w896:i16)
            n579 = Boolean To (0,1)(Boolean="Convolution") -> (0, 1=w904:i16)
            n580 = script code="frames(f).gain             = gain;\n   frames(f).threshold    = threshold;\n   frames(f).brightness   = brightness;\n   frames(f).convOpt      = convOpt;\n   frames(f).maskOpt      = maskOpt;\n   frames(f).maskSize      = maskSize;\n   frames(f).maskShiftX   = maskShiftX;\n   frames(f).maskShiftY   = maskShiftY;\n\n     processObject;\n\n   objProZ = frames(f).objPro(:,:,zInd);"("gain"="Gain", "threshold"="Threshold", "brightness"="Brigtness", "convOpt"=w904, "maskSize"="Mask size (%)", "maskShiftX"="Mask Shift X", "maskShiftY"="Mask Shift Y", "maskOpt"=w896) -> ("??"=w905:errorcluster)  [unwired: 1 in, 1 out]
          }
          event "Left": Mouse Down {
            n581 = event-data() -> ()  [unwired: 1 in, 7 out]
            n582 = global read "callback_Done.vi" "X Motor Reference"() -> (w906:refnum<k7>)
            n583 = invoke class="MG17Motor" method="MoveJog"(reference=w906, "lChanID"=0, "lJogDir"=2147483647) -> ()  [unwired: 2 in, 5 out]
          }
          event "Right": Mouse Down {
            n584 = event-data() -> ()  [unwired: 1 in, 7 out]
            n585 = global read "callback_Done.vi" "X Motor Reference"() -> (w909:refnum<k7>)
            n586 = invoke class="MG17Motor" method="MoveJog"(reference=w909, "lChanID"=0, "lJogDir"=0) -> ()  [unwired: 2 in, 5 out]
          }
          event "Up": Mouse Down {
            n587 = event-data() -> ()  [unwired: 1 in, 7 out]
            n588 = global read "callback_Done.vi" "Y Motor Reference"() -> (w914:refnum<k7>)
            n589 = invoke class="MG17Motor" method="MoveJog"(reference=w914, "lChanID"=0, "lJogDir"=2147483647) -> ()  [unwired: 2 in, 5 out]
          }
          event "Down": Mouse Down {
            n590 = event-data() -> ()  [unwired: 1 in, 7 out]
            n591 = global read "callback_Done.vi" "Y Motor Reference"() -> (w917:refnum<k7>)
            n592 = invoke class="MG17Motor" method="MoveJog"(reference=w917, "lChanID"=0, "lJogDir"=0) -> ()  [unwired: 2 in, 5 out]
          }
          event "FocusUp": Mouse Down {
            n593 = event-data() -> ()  [unwired: 1 in, 7 out]
            n594 = global read "callback_Done.vi" "Z Motor Reference"() -> (w920:refnum<k7>)
            n595 = invoke class="MG17Motor" method="MoveJog"(reference=w920, "lChanID"=0, "lJogDir"=0) -> ()  [unwired: 2 in, 5 out]
          }
          event "FocusDown": Mouse Down {
            n596 = event-data() -> ()  [unwired: 1 in, 7 out]
            n597 = global read "callback_Done.vi" "Z Motor Reference"() -> (w923:refnum<k7>)
            n598 = invoke class="MG17Motor" method="MoveJog"(reference=w923, "lChanID"=0, "lJogDir"=2147483647) -> ()  [unwired: 2 in, 5 out]
          }
          event "Left", "Right": Mouse Up {
            n599 = event-data() -> ()  [unwired: 1 in, 7 out]
            n600 = global read "callback_Done.vi" "X Motor Reference"() -> (w924:refnum<k7>)
            n601 = invoke class="MG17Motor" method="StopImmediate"(reference=w924, "lChanID"=0) -> ()  [unwired: 2 in, 4 out]
          }
          event "Up", "Down": Mouse Up {
            n602 = event-data() -> ()  [unwired: 1 in, 7 out]
            n603 = global read "callback_Done.vi" "Y Motor Reference"() -> (w927:refnum<k7>)
            n604 = invoke class="MG17Motor" method="StopImmediate"(reference=w927, "lChanID"=0) -> ()  [unwired: 2 in, 4 out]
          }
          event "FocusUp", "FocusDown": Mouse Up {
            n605 = event-data() -> ()  [unwired: 1 in, 7 out]
            n606 = global read "callback_Done.vi" "Z Motor Reference"() -> (w929:refnum<k7>)
            n607 = invoke class="MG17Motor" method="StopImmediate"(reference=w929, "lChanID"=0) -> ()  [unwired: 2 in, 4 out]
          }
          event "LightValue (v)": Value Change {
            n608 = event-data() -> ()  [unwired: 1 in, 6 out]
            n609 = call <userlib>:"U3 eDAC Example.vi"("Voltage"="LightVoltage") -> ()  [unwired: 10 in, 1 out]
          }
          event "Light On (5v)": Value Change {
            n610 = event-data() -> ()  [unwired: 1 in, 6 out]
            n611 = call <userlib>:"U3 eDAC Example.vi"("Voltage"=5.0) -> ()  [unwired: 10 in, 1 out]
          }
          event "Light Off (0v)": Value Change {
            n612 = event-data() -> ()  [unwired: 1 in, 6 out]
            n613 = call <userlib>:"U3 eDAC Example.vi"("Voltage"=0.0) -> ()  [unwired: 10 in, 1 out]
          }
          event User Event {
            n614 = event-data() -> ("Event"=w934:u32)  [unwired: 1 in, 3 out]
            n615 = case shown="4" w934 {
              tunnel: w933 -> [w961 _]
              frame 4 {
                # "ShowVideo"
                n616 = global read "GlobalVariables.vi" "Toup Resolution"() -> (w949:cluster{"pWidth":i32, "pHeight":i32})
                n617 = Unbundle By Name("Toup Crop 5440x3648") -> ("Horizontal Offset"=w943:i32, "Vertical Offset"=w946:i32, "Horizontal Width"=w942:i32, "Vertical Width"=w945:i32)
                n618 = Unbundle(w949) -> ("pWidth"=w956:i32, "pHeight"=w955:i32)
                n619 = Multiply(x=w956, y=w955) -> (x*y=w959:i32)
                n620 = global read "GlobalVariables.vi" "Toup Temp Img"() -> (w951:T5)
                n621 = Initialize Array(u32 0, w959) -> (w957:u32[])
                n622 = Add(x=w946, y=w945) -> (x+y=w947:i32)
                n623 = Add(x=w943, y=w942) -> (x+y=w944:i32)
                n624 = Build Array(w943, w946, w944, w947) -> (w940:i32[])
                n625 = local read "Camera Idx"() -> (w939:i32)
                n626 = global read "GlobalVariables.vi" "Toup Ref Img"() -> (w950:T5)
                n627 = dll-call lib="D:/amcamsdk.20210816/extras/labview/toupcam.dll" fn="Toupcam_PullImage"("htoupcam"=w961, "pImageData"=w957, "bits"=32, "nWidth"=w956, "nHeight"=w955) -> ("pImageData"=w960:u32[])  [unwired: 8 in, 2 out]
                n628 = Reshape Array(w960, w955, w956) -> (w953:u32[][])
                n629 = call "IMAQ ArrayToColorImage"("Image Pixels (U32)"=w953, "Image"=w951) -> ("Image Out"=w948:T5)  [unwired: 3 in, 1 out]
                n630 = call "IMAQ ExtractSingleColorPlane"("Color Plane"="Color Plane", "Image Dst"=w950, "Image Src"=w948) -> ("Image Dst Out"=w936:T5)  [unwired: 7 in, 1 out]
                n631 = call "IMAQ ImageToArray"("Optional Rectangle"=w940, "Image"=w936) -> ("Image Pixels (U8)"=w938:u8[][])  [unwired: 2 in, 4 out]
                n632 = case shown="0, Default" w939 {
                  tunnel: w938 -> [w964 w966]
                  tunnel: [w964 w965] -> w937
                  frame 0, Default {
                  }
                  frame 1 {
                    n633 = Transpose 2D Array(2D array=w966) -> (transposed array=w967:u8[][])
                    n634 = for {
                      tunnel: w967 -> [w969] mode=indexing
                      tunnel: [w968] -> w965 mode=indexing
                      n635 = Reverse 1D Array(array=w969) -> (reversed array=w968:u8[])
                    }
                  }
                }
                n636 = property on="objRef" class="IntGraph (strict)"("Value"=w937) -> ()  [unwired: 2 in, 2 out]
                n637 = case shown="True" "Full Toup Resolution" {
                  tunnel: w936 -> [_ w963]
                  frame False {
                  }
                  frame True {
                    n638 = call "IMAQ ImageToArray"("Image"=w963) -> ("Image Pixels (U8)"=→"Image 2":u8[][])  [unwired: 3 in, 4 out]
                  }
                }
              }
              frame 0, Default {
              }
            }
          }
          event "Expotime (ms)": Value Change {
            n639 = event-data() -> ()  [unwired: 1 in, 5 out]
            n640 = Multiply(x="Expotime (ms)", y=u32 1000) -> (x*y=w970:dbl)
            n641 = dll-call lib="D:/amcamsdk.20210816/extras/labview/toupcam.dll" fn="Toupcam_put_ExpoTime"("htoupcam"=w973, "Expotime"=w970) -> ()  [unwired: 6 in, 2 out]
          }
          event "ExpoGain": Value Change {
            n642 = event-data() -> ()  [unwired: 1 in, 5 out]
            n643 = dll-call lib="D:/amcamsdk.20210816/extras/labview/toupcam.dll" fn="Toupcam_put_ExpoAGain"("htoupcam"=w974, "ExpoGain"="ExpoGain") -> ()  [unwired: 6 in, 2 out]
          }
          event "Brightness", "Contrast", "Gamma", "Hue", "Saturation": Value Change {
            n644 = event-data() -> ()  [unwired: 1 in, 5 out]
            n645 = dll-call lib="D:/amcamsdk.20210816/extras/labview/toupcam.dll" fn="Toupcam_put_Brightness"("htoupcam"=w976, "Brightness"="Brightness") -> ("htoupcam"=w982:i32)  [unwired: 5 in, 2 out]
            n646 = dll-call lib="D:/amcamsdk.20210816/extras/labview/toupcam.dll" fn="Toupcam_put_Contrast"("htoupcam"=w976, "Contrast"="Contrast") -> ()  [unwired: 6 in, 2 out]
            n647 = dll-call lib="D:/amcamsdk.20210816/extras/labview/toupcam.dll" fn="Toupcam_put_Gamma"("htoupcam"=w976, "Gamma"="Gamma") -> ()  [unwired: 6 in, 2 out]
            n648 = dll-call lib="D:/amcamsdk.20210816/extras/labview/toupcam.dll" fn="Toupcam_put_Hue"("htoupcam"=w982, "Hue"="Hue") -> ()  [unwired: 6 in, 2 out]
            n649 = dll-call lib="D:/amcamsdk.20210816/extras/labview/toupcam.dll" fn="Toupcam_put_Saturation"("htoupcam"=w982, "Saturation"="Saturation") -> ()  [unwired: 6 in, 2 out]
          }
          event "Camera Idx": Value Change {
            n650 = event-data() -> ()  [unwired: 1 in, 5 out]
          }
          event "Calculate Shrink": Value Change {
            n651 = event-data() -> ()  [unwired: 1 in, 6 out]
            n652 = local read "Start Time"() -> (w990:timestamp)
            n653 = Get Date/Time In Seconds() -> (seconds since 1Jan1904=w991:timestamp)
            n654 = local read "Shrink"() -> (w985:dbl)
            n655 = Subtract(x=w991, y=w990) -> (x-y=w989:dbl)
            n656 = Subtract(x=w985, y=0.01) -> (x-y=w984:dbl)
            n657 = Divide(x=w984, y=w989) -> (x/y=w988:dbl)
            n658 = Divide(x=w988, y=86400.0) -> (x/y=→"CalculatedRate":dbl)
          }
        }
        n659 = call <vilib>:"Simple Error Handler.vi"("type of dialog (OK msg:1)"=w755, "error in (no error)"=w754) -> ()  [unwired: 3 in, 5 out]
      }
      n660 = while {
        stop <- FALSE stop-if-true
        n661 = case shown="True" "StartShrinking" {
          frame False {
          }
          frame True {
            n662 = local read "Shrink"() -> (w79:dbl)
            n663 = Wait (ms)(milliseconds to wait=u32 60000) -> ()  [unwired: 1 out]
            n664 = Divide(x="ShrinkRate(mm/day)", y=1440.0) -> (x/y=w78:dbl)
            n665 = Add(x=w78, y=w79) -> (x+y=w77:dbl)
            n666 = local write "Shrink"(w77) -> ()
          }
        }
      }
    }
    frame Error {
      w992 = T6 1 items=["no dialog", "OK message", "continue or stop message", "OK message + warnings", "continue/stop + warnings"] ("type of dialog (OK msg:1)")
      n667 = call <vilib>:"Simple Error Handler.vi"("type of dialog (OK msg:1)"=w992, "error in (no error)"=w993) -> ()  [unwired: 3 in, 5 out]
    }
  }
